vi "CMSClient.vi"() -> ()   [LabVIEW 2013]
uses:
  Controls/CMS Win8 Cluster.ctl
  Controls/CMS Win4 Cluster.ctl
  Controls/DB - Logon Info.ctl
  Controls/DB - Logon Extra Info.ctl
  Controls/Enum - CMS State.ctl
  <vilib>/Utility/miscctls.llb/LVPointTypeDef.ctl
  Controls/CMS Windows Tab.ctl
  Controls/DB - CMS Config WindowView.ctl
  Controls/DB - CMS Execute Active Process.ctl
  Controls/DB - Config WindowView Enum.ctl
  Controls/DB - [Execute].[ActiveProcess] Enum.ctl
  Controls/Global CMS.vi
  <vilib>/Utility/config.llb/Write Key (String).vi
  <vilib>/regexp/Match Regular Expression.xnode
  Controls/Message Code - Enum.ctl
  Controls/Enum - SRTRS State.ctl
  <vilib>/Utility/config.llb/NI_LVConfig.lvlib
panel:
  in  "Tab Footer":enum32{"Page 1"}(tab) caption="Tab Header"
  out "Date Time":string="ver. 13" caption="Plant and Furnace Name"
  in  "Tab Header":enum32{"Page 1"}(tab)
  out "LogoName":picture
  in  "Close":bool
  out "Plant and Furnace Name":string="ver. 13"
  out "ApplicationName":string caption="[LogoName]"
  in  "Tab Body":T1(tab)
  out "Cluster7 WIN8":T2 {"% Hold Complete" scale=0.0..100.0}
  out "Cluster6 WIN8":T2 {"% Hold Complete" scale=0.0..100.0}
  out "Cluster5 WIN8":T2 {"% Hold Complete" scale=0.0..100.0}
  out "Cluster4 WIN8":T2 {"% Hold Complete" scale=0.0..100.0}
  out "Cluster3 WIN8":T2 caption="Cluster3" {"% Hold Complete" scale=0.0..100.0}
  out "Cluster2 WIN8":T2 caption="Cluster2" {"% Hold Complete" scale=0.0..100.0}
  out "Cluster1 WIN8":T2 {"% Hold Complete" scale=0.0..100.0}
  out "Cluster0 WIN8":T2 {"% Hold Complete" scale=0.0..100.0}
  out "Cluster3 WIN4":T3={"Bay"="", "Seq Status"="Waiting to Start", "Record"="", "Hold"="", "% Hold Complete"=0, "Alarm"="", "Temperature"="", "Units"="", "Graph"=[], "Last Updated On"="", "Current Window"=FALSE, "[PlantId.SystemId]"="", "Last Updated (Local)"=""} {"% Hold Complete" scale=0.0..100.0}
  out "Cluster2 WIN4":T3={"Bay"="", "Seq Status"="Waiting to Start", "Record"="", "Hold"="", "% Hold Complete"=0, "Alarm"="", "Temperature"="", "Units"="", "Graph"=[], "Last Updated On"="", "Current Window"=FALSE, "[PlantId.SystemId]"="", "Last Updated (Local)"=""} {"% Hold Complete" scale=0.0..100.0}
  out "Cluster1 WIN4":T3={"Bay"="", "Seq Status"="Waiting to Start", "Record"="", "Hold"="", "% Hold Complete"=0, "Alarm"="", "Temperature"="", "Units"="", "Graph"=[], "Last Updated On"="", "Current Window"=FALSE, "[PlantId.SystemId]"="", "Last Updated (Local)"=""} {"% Hold Complete" scale=0.0..100.0}
  out "Cluster0 WIN4":T3={"Bay"="", "Seq Status"="Waiting to Start", "Record"="", "Hold"="", "% Hold Complete"=0, "Alarm"="", "Temperature"="", "Units"="", "Graph"=[], "Last Updated On"="", "Current Window"=FALSE, "[PlantId.SystemId]"="", "Last Updated (Local)"=""} {"% Hold Complete" scale=0.0..100.0}
  out "Last Updated On":string="2014-10-23 15:23" caption="last updated:"
  out "Key Values":T4={"Recording Duration"=1440.0, "Remaining Hold Time"=1620.0, "Current Temp"=79.84, "Key Values Temperature Units"="°C"} {"Current Temp" format="%#_4f"; "Remaining Hold Time" format="%<%H:%M>t"; "Recording Duration" format="%<%H:%M:%S>t"}
  out "Chart":dynamicdata(graph)
  out "TransactionRunNo (Execute)":string="12" caption="Run No."
  out "cRIO Status":string="DAQ Started. cRIO Simulate Mode." caption="Data Logger"
  out "Transaction No (Execute)":string="110" caption="Transaction No."
  out "% Hold. Time Completed":dbl(slide)=10.0 scale=0.0..100.0
  out "Process Completed":bool
  out "Hold Time Completed":bool
  out "ET3504 Status":string="Program [33]. Segment [Dwell]. Program Status [Running]. ET3500 Simulate Mode." caption="Furnace"
  out "Sequence Status":string="Seq 1/2: +150°C/hr to 80°C & Holding for 00:30 (hh:mm)" caption="Sequence"
  out "Overall Status":bool
  out "WIN1 Bay":string="SRSB-B2"
  in  "MyTab":T5(tab)
  out "Skip Timer Count":i32
  out "WindowView (ORDERed by DB)":string[][](array[string])=[["WIN8", "0", "30", "2", "-1", "0", "4070.SRSB-A1", "4070.SRSB-B2", "4070.SRSB-C3", "4070.SRSB-D4", "4070.SRSB-E5", "4070.SRSB-F6", "4070.SRSB-G7", "4070.SRSB-H8", "", "", "", "", "", "", "", "", "", "", "", ""], ["WIN1", "1", "30", "2", "-1", "0", "4070.SRSB-A1", "4070.SRSB-B2", "4070.SRSB-C3", "4070.SRSB-D4", "4070.SRSB-E5", "", "", "", "", "", "", "", "", "", "", "", "", "", "", ""], ["WIN4", "3", "10", "2", "-1", "0", "4070.SRSB-A1", "4070.SRSB-B2", "", "4070.SRSB-D4", "4070.SRSB-E5", "", "", "", "", "", "", "", "", "", "", "", "", "", "", ""]]
  out "[ToggleWinInterval] Timer":dbl=1.201359748840332 format="%.1g"
  out "[ToggleTabInterval] Timer":dbl=10.53461217880249 format="%.1g"
  out "Current [TabId]":string="WIN8"
  out "[TabId] Index":i32
  out "Time (WIN8 Click)":u32
  out "WIN8 IQ":i32
  out "WIN4 IQ":i32
  out "[ToggleTab] Override":bool=TRUE
  out "[ToggleTab]":bool=TRUE
  out "Page Label when Menu is Clicked":string="WIN8"
  out "New [TabId] Index":i32
  out "Reset [TabId] Index":bool
  out "Stay in [WINDOWxx]":bool
  out "[WINDOWxx] Stay":string="4070.SRSB-A1"
  out "[WINDOWxx]":string="4070.SRSB-C3"
  out "Empty [WINDOWxx]":string[](array[string])
  out "Skip WIN Timer":bool=TRUE
  out "Skip TAB Timer":bool=TRUE
  out "Current WindowView":string[](array[string])
  out "# of requested Windowxx":i32
  out "Property Node":errorcluster
  out "Load History":errorcluster
  out "Cluster0 WIN1":T2={"Bay"="", "Seq Status"="Waiting to Start", "Record"="", "Hold"="", "% Hold Complete"=0, "Alarm"="", "Temperature"="", "Units"="", "Graph"=[], "Last Updated On"="", "Current Window"=FALSE, "[PlantId.SystemId]"="", "Last Updated (Local)"=""} {"% Hold Complete" scale=0.0..100.0}
  out "SubPanel Error":errorcluster
  out "Logon OK":bool
  in  "[TabUserAccess]":bool[](array[boolean])=[FALSE, FALSE, FALSE, FALSE, FALSE, FALSE, FALSE, FALSE, FALSE, FALSE, FALSE, FALSE, FALSE, FALSE, FALSE, FALSE, FALSE, FALSE, FALSE, FALSE]
  in  "Logon Extra":T6
  in  "Logon":T7
  out "Current VI's path":path=path "C:/Users/CK/workspace/LabVIEW/Stress Relief Temperature Recording/VIs/CMSClient.vi"
  out "Front Panel Window:State":T8(ring)=enum."Closed"
  out "Execution:State":T9(ring)=enum."Idle"
  out "Admin User UI":refnum<vi>
  out "Logon UI":refnum<vi>
  out "Config UI":refnum<vi>
  in  "Application":string="CMS"
  out "ini File":errorcluster
  out "LogonName Error":errorcluster
  out "[ToggleTabInterval]":dbl=10.0 format="%#_13g"
  out "Min [ToggleWinInterval]":i32=2
  out "Station":string="C001"
  out "Plant":string="4070"
  out "[ToggleWinInterval]":dbl=2.0 format="%#_13g"
  out "Min [ToggleTabInterval]":i32=10
  out "LabVIEW Directory Path":path=path "C:/Program Files (x86)/National Instruments/LabVIEW 2013"
  out "Application:Name":string="LabVIEW.exe"
  out "[TimeZone] (Plant)":string="+8"
  out "[CmsServerTz] (CMS)":string="+7"
  out "TimeZone Diff (NA)":i32=-1
  out "Time Offset":dbl=-0.44188642501831055
  out "Plant and Furnace Name (B4 Logon)":string="ver. 13" caption="Plant and Furnace Name"
  out "DisplayDurationInMin":i32=60
  out "Error Out":errorcluster
  out "Show Debug TAB":bool=TRUE caption="Show Debug Tab"
  out "Lite Version":bool
  out "Quit Flag":bool=TRUE
  out "Close Flag":bool=TRUE
  out "WIN8 Array":refnum<vi>[](array[refnum])
  out "WIN4 Array":refnum<vi>[](array[refnum])
  in  "PlantId.SystemId - Last Updated (Local)":string[][](array[string])
  out "MHandler":errorcluster
  out "DB":errorcluster
  in  "DB - Logon":bool=TRUE
  out "File Version":string="ver. 13.0f1"
  in  "Debug Close":bool caption="Close"
  # "Process Status"
  # "System Status"
  # "(hh:mm:ss)"
  # "(hh:mm)"
  # "User Details"
  # "System Status"
  # "Logon"
  # "2014-10-21 15:01\n[TabId],                         w.[IsDefault],        v.[ToggleTabInterval],w.[ToggleWinInterval], v.[ToggleTab],        v.[DisplayPlant],       w.[Window01],            w.[Window02]"
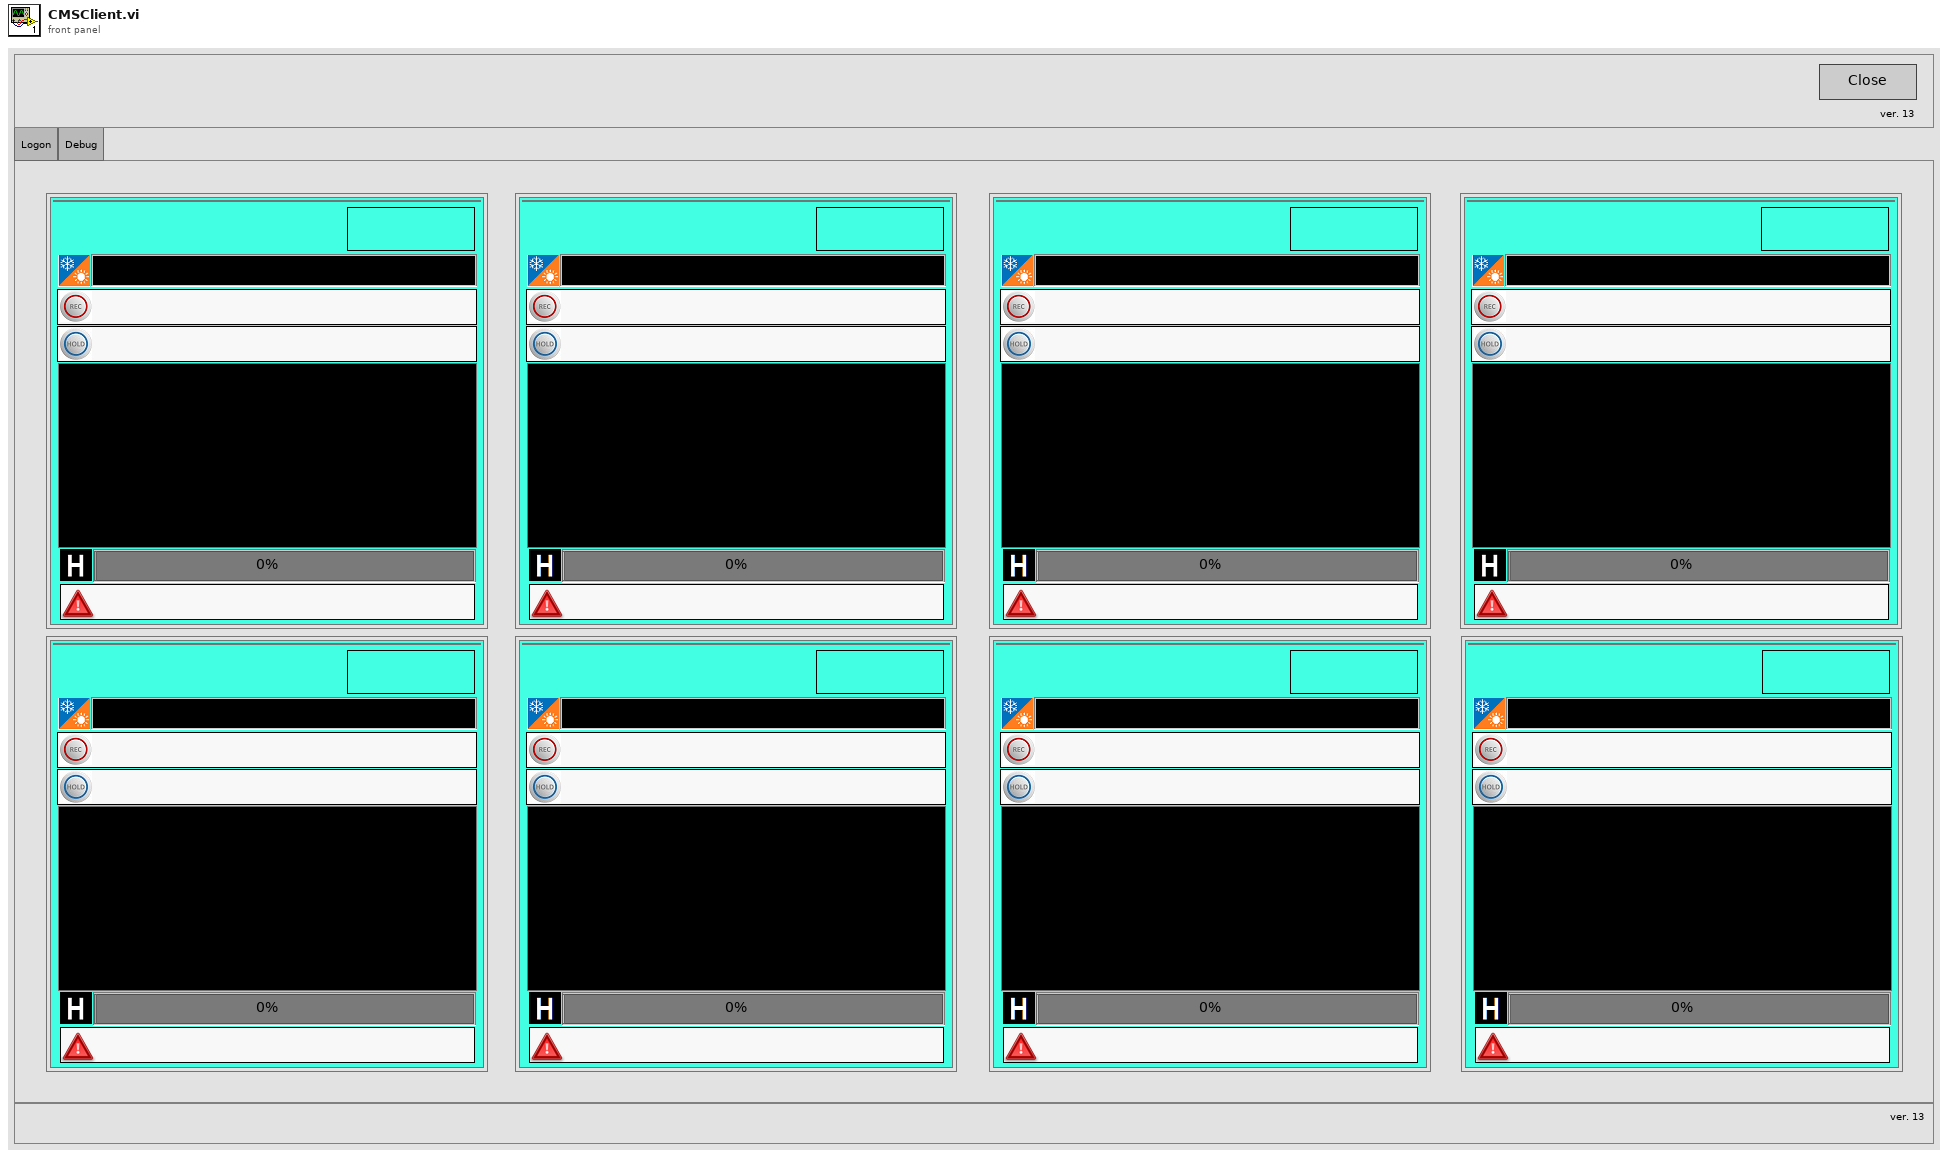
[diagram p1: front panel]
types:
  T1 = enum32{"WIN8", "WIN4", "WIN1", "Admin", "Config", "Logon", "Debug"}
  T2 = typedef "CMS Win8 Cluster.ctl" = cluster{"Bay":string, "Seq Status":string, "Record":string, "Hold":string, "% Hold Complete":u8, "Alarm":string, "Temperature":string, "Units":string, "Graph":dbl[][], "Last Updated On":string, "Current Window":bool, "[PlantId.SystemId]":string, "Last Updated (Local)":string}
  T3 = typedef "CMS Win4 Cluster.ctl" = cluster{"Bay":string, "Seq Status":string, "Record":string, "Hold":string, "% Hold Complete":u8, "Alarm":string, "Temperature":string, "Units":string, "Graph":dbl[][], "Last Updated On":string, "Current Window":bool, "[PlantId.SystemId]":string, "Last Updated (Local)":string}
  T4 = cluster{"Recording Duration":dbl, "Remaining Hold Time":dbl, "Current Temp":dbl, "Key Values Temperature Units":string}
  T5 = enum32{"WindowView", "Single Window", "SubPanel", "Settings", "Others", "DB"}
  T6 = typedef "DB - Logon Extra Info.ctl" = cluster{"Plant Name":string, "UserName":string, "Hostname [ClientName]":string, "IsUnicode":bool}
  T7 = typedef "DB - Logon Info.ctl" = cluster{"PlantID":string, "SystemID":string, "UserID":string, "DomainID":string, "LanguageID":string, "StationID":string}
  T8 = enum32{"Invalid", "Standard", "Closed", "Hidden", "Minimized", "Maximized"}
  T9 = enum32{"Bad", "Idle", "Run top level", "Running"}
  T10 = typedef "Enum - CMS State.ctl" = enum16{"READY TO START", "RUNNING Process", "QUIT"}
  T11 = enum16{"Always On", "Always Off", "Off While Running"}
  T12 = typedef "CMS Windows Tab.ctl" = enum32{"WIN8", "WIN4", "WIN1", "Admin", "Config", "Logon", "Debug"}
  T13 = typedef "LVPointTypeDef.ctl" = cluster{"Horizontal":i16, "Vertical":i16}
  T14 = enum8{"Enabled", "Disabled", "Disabled and Grayed Out"}
  T15 = cluster{"LogoFile":string, "Software Solution Name":string}
  T16 = typedef "Connection Information Cluster.ctl" = cluster{"Connection ":string, "Username":string, "Password":string}
  T17 = cluster{"Show LabVIEW Error":bool, "Show Debug Tab":bool, "Show Scrollbars":bool, "ToggleTab":bool}
  T18 = typedef "imagedata.ctl" = cluster{"image type":i32, "image depth":i32, "image":u8[], "mask":u8[], "colors":u32[], "Rectangle":cluster{"left":i16, "top":i16, "right":i16, "bottom":i16}}
  T19 = typedef "Enum - SRTRS State.ctl" = enum16{"READY TO START", "START Recipe", "START Recovery", "BEGIN Process", "RUNNING Process", "END Process", "Spare Enum", "END Recipe", "ERROR Handling", "QUIT"}
  T20 = typedef "DB - CMS Config WindowView.ctl" = enum16{"SELECT [Config].[View]"}
  T21 = typedef "DB - Config WindowView Enum.ctl" = enum16{"w.[TabId]", "w.[Number]", "w.[ToggleTabInterval]", "w.[ToggleWinInterval]", "v.[ToggleTab]", "v.[DisplayPlant]", "w.[Window01]", "w.[Windowxx]"}
  T22 = typedef "DB - CMS Execute Active Process.ctl" = enum16{"INSERT INTO [Execute].[ActiveProcess]", "UPDATE [Execute].[ActiveProcess]", "SELECT [Execute].[ActiveProcess]", "UPDATE FILESTREAM", "SELECT FILESTREAM", "Check [IsActive]"}
  T23 = typedef "DB - [Execute].[ActiveProcess] Enum.ctl" = enum16{"[IsActive]", "[TransactionNo]", "[TransactionRunNo]", "[SequenceStatus]", "[StartRecordTime]", "[EndRecordTime]", "[StartHoldTime]", "[EndHoldTime]", "[Message1]", "[Message2]", "[HoldTimeRemaining]", "[HoldTimePercentage]", "[HoldProgressColor]", "[OrderNumbers]", "[CurrentTemp]", "[UnitOfTemperature]", "[IsAppClientLive]", "[RawDataFile]", "[RecordedMinutes]", "[FurnaceControlStatus]", "[FurnaceControlColor]", "[ControllerStatus]", "[ControllerColor]", "[IsControllerOnline]", "[ProcessColor]", "[OverallColor]", "[LastUpdatedOn]", "[LastUpdatedCmsTime]", "[Inactive]"}
  T24 = enum16{"INSERT INTO [Execute].[ActiveProcess]", "UPDATE [Execute].[ActiveProcess]", "SELECT [Execute].[ActiveProcess]", "UPDATE FILESTREAM", "SELECT FILESTREAM"}
  T25 = typedef "NI_LVConfig.lvlib/Config Data RefNum.ctl" = refnum<k1>
  T26 = typedef "Message Code - Enum.ctl" = enum16{"<APP><I 100>", "<APP><E 101>", "<APP><I 110>", "<APP><W 111>", "<APP><I 112>", "<APP><W 113>", "<APP><I 114>", "<APP><I 115>", "<APP><I 116>", "<APP><W 117>", "<APP><I 120>", "<APP><W 121>", "<APP><E 122>", "<APP><W 130>", "<APP><W 131>", "<APP><W 132>", "<APP><W 133>", "<APP><W 134>", "<DB><I 150>", "<DB><I 151>", "<DB><W 152>", "<APP><I 200>", "<APP><I 201>", "<APP><W 202>", "<APP><E 203>", "<DB><I 300>", "<DB><I 301>", "<DB><W 302>", "<DB><I 305>", "<DB><I 306>", "<DB><W 307>", "<DB><W 310>", "<cRIO><I 400>", "<cRIO><W 401>", "<cRIO><I 402>", "<cRIO><W 403>", "<ET><I 500>", "<ET><W 501>", "<ET><I 600>", "<ET><W 601>", "<ET><E 602>", "<ET><I 610>", "<ET><W 611>", "<ET><E 612>"}
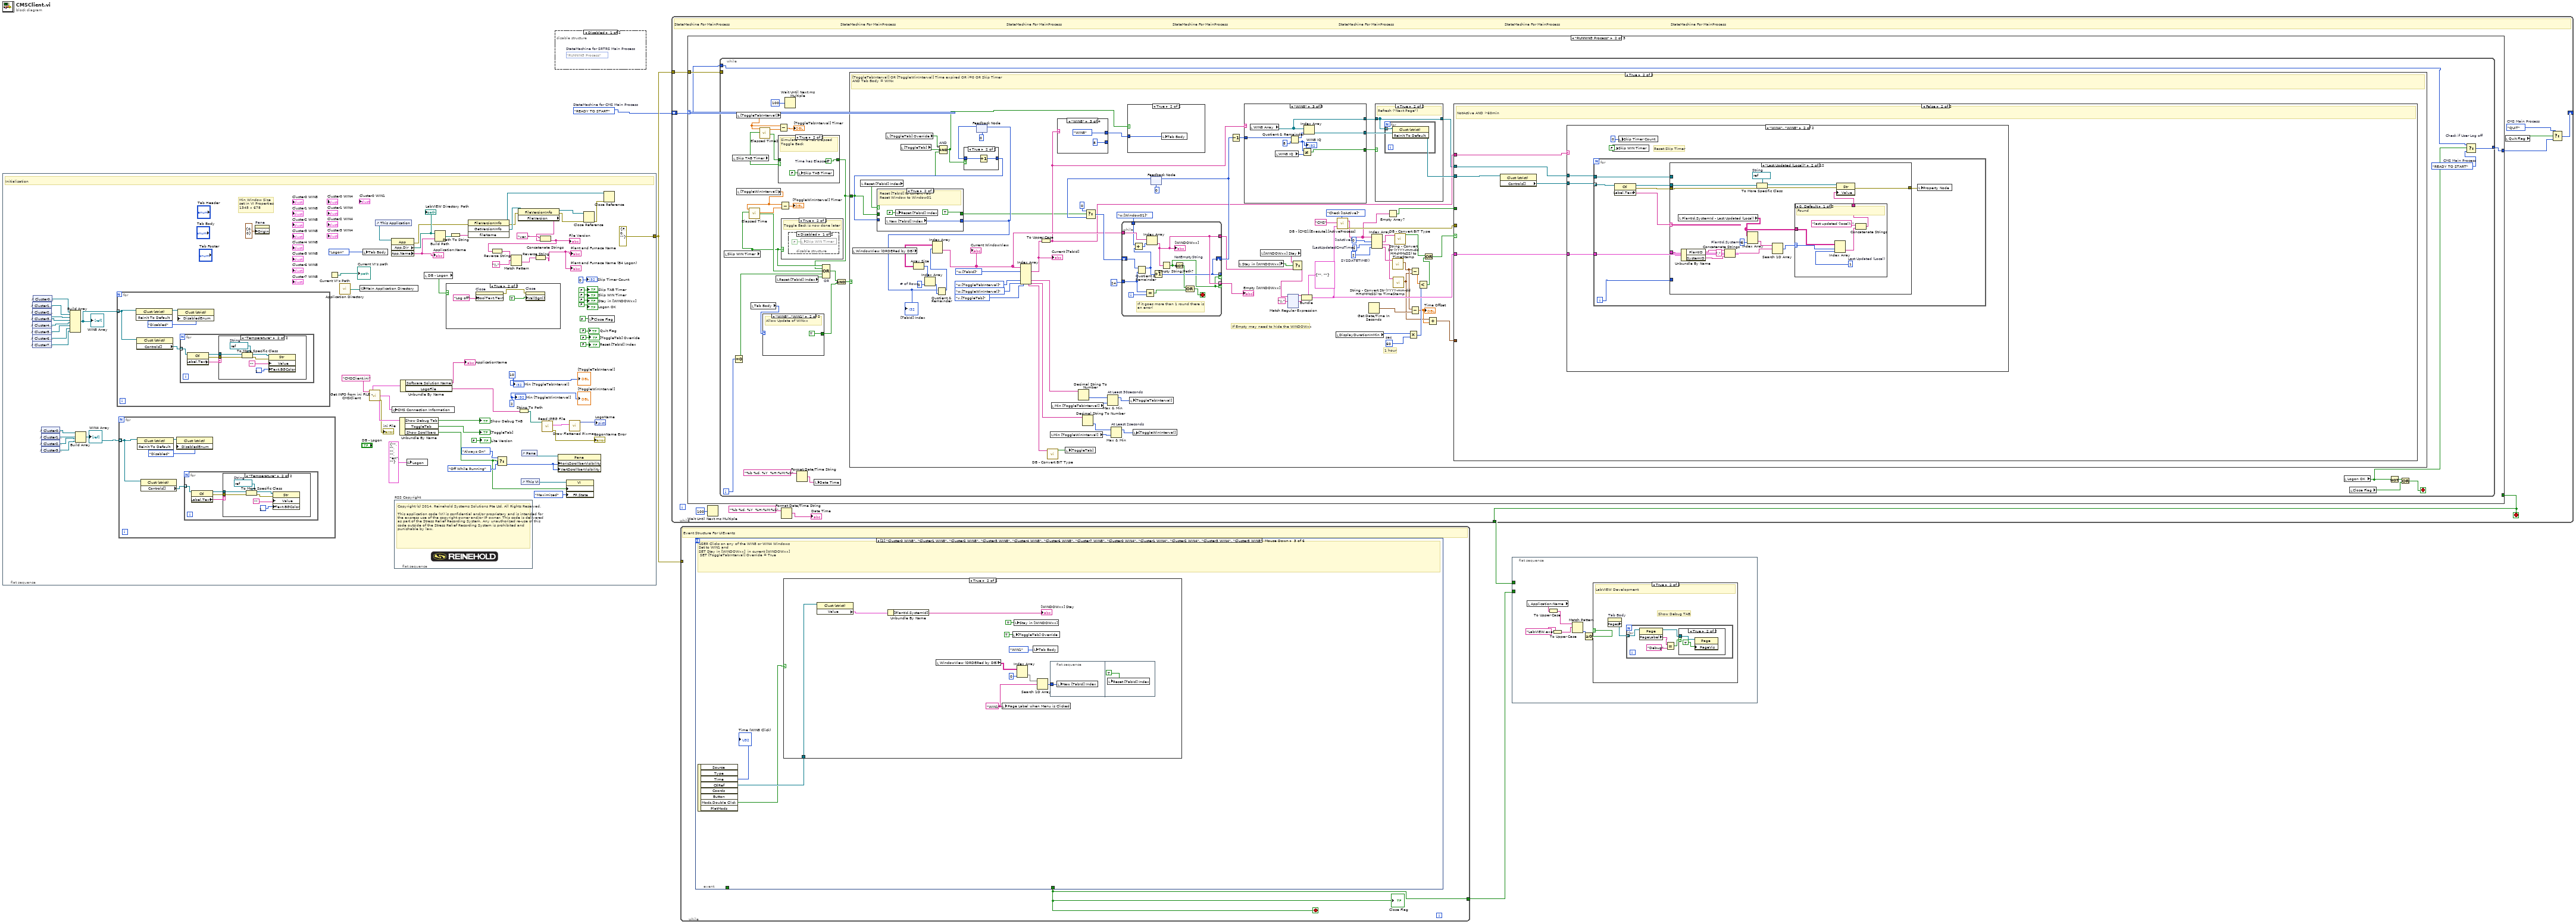
[diagram p0: block diagram]
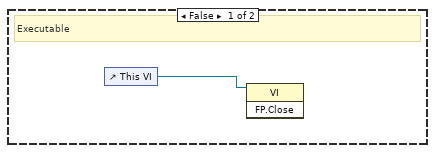
[diagram p2: hidden frame]
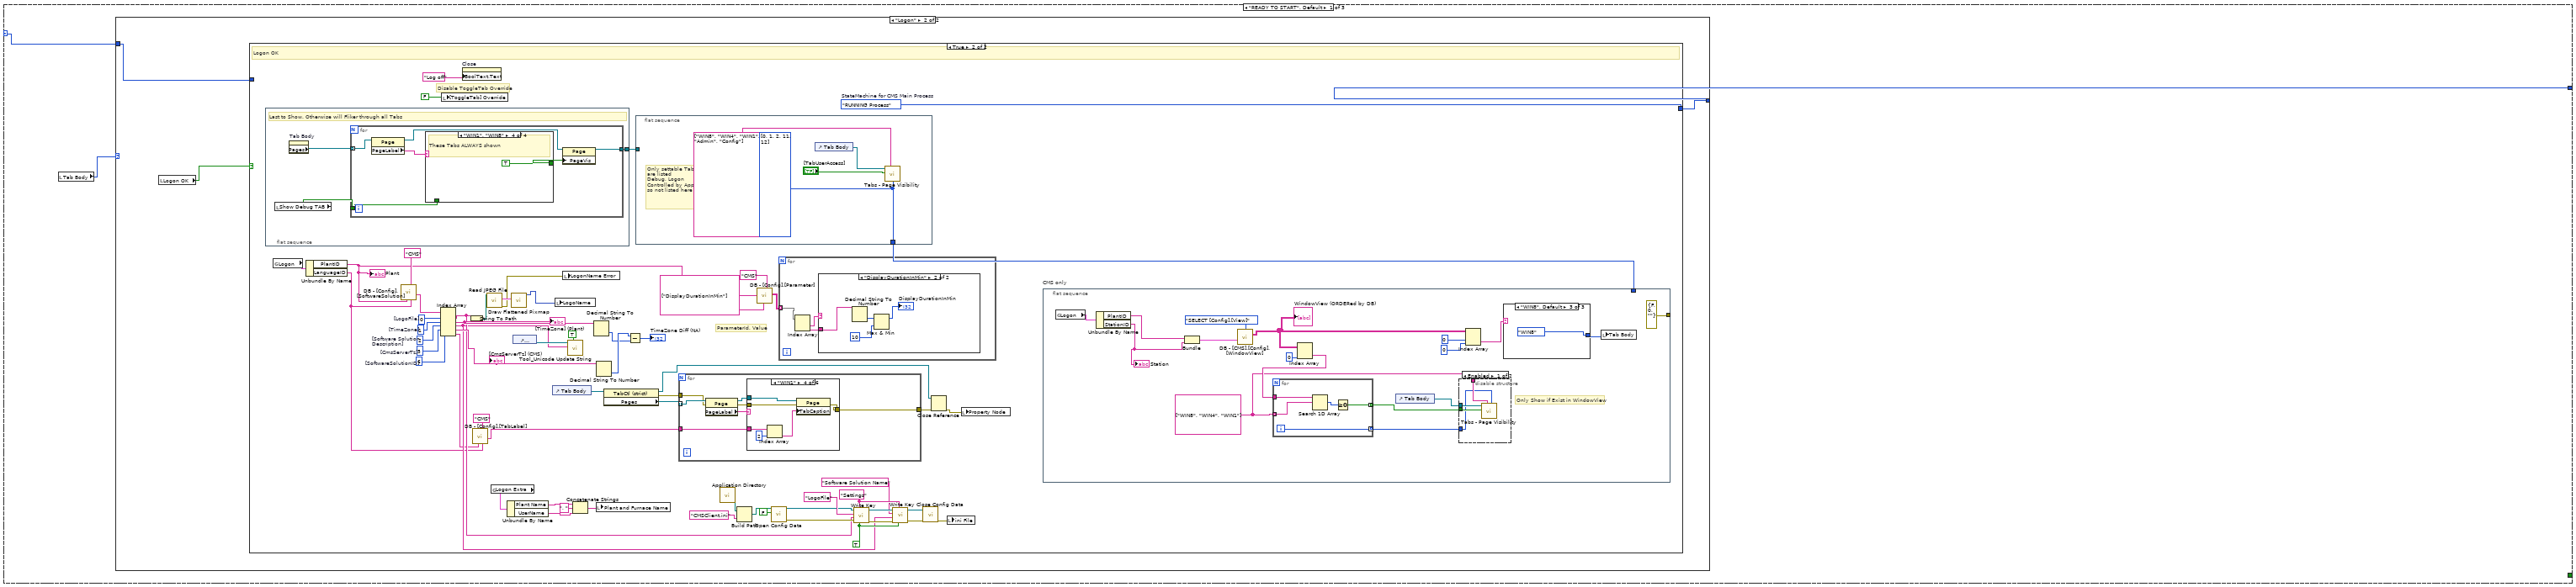
[diagram p5: hidden frame]
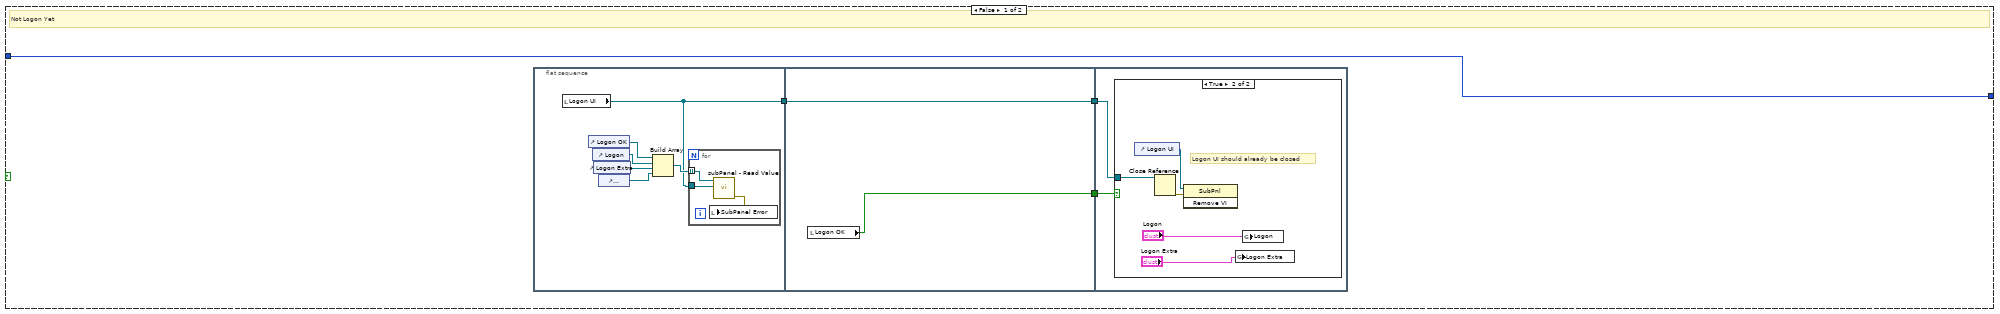
[diagram p7: hidden frame]
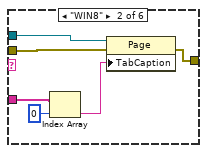
[diagram p11: hidden frame]
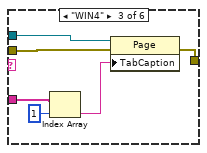
[diagram p12: hidden frame]
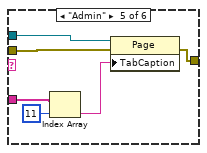
[diagram p13: hidden frame]
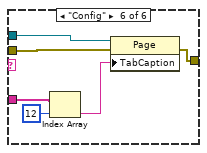
[diagram p14: hidden frame]
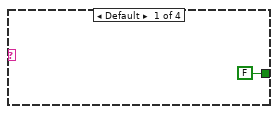
[diagram p15: hidden frame]
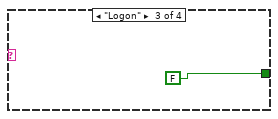
[diagram p17: hidden frame]
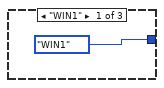
[diagram p19: hidden frame]
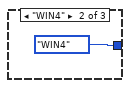
[diagram p20: hidden frame]
diagram:
  w3 = Enum_-_CMS_State."READY TO START"  # StateMachine for CMS Main Process
  n1 = flat-sequence {
    tunnel: [errorcluster {"status"=FALSE, "code"=0, "source"=""} ("error constant")] -> w4
    frame #0 {
      w8 = 2
      w9 = 10
      # "Min Window Size\nset in VI Properties\n1345 x 678"
      # "Initialisation"
      n2 = control-ref of="Cluster1 WIN8"() -> (w67:refnum<vi>)
      n3 = control-ref of="Cluster2 WIN8"() -> (w68:refnum<vi>)
      n4 = control-ref of="Cluster3 WIN8"() -> (w69:refnum<vi>)
      n5 = control-ref of="Cluster4 WIN8"() -> (w70:refnum<vi>)
      n6 = control-ref of="Cluster5 WIN8"() -> (w71:refnum<vi>)
      n7 = control-ref of="Cluster6 WIN8"() -> (w72:refnum<vi>)
      n8 = control-ref of="Cluster7 WIN8"() -> (w73:refnum<vi>)
      n9 = control-ref of="Cluster0 WIN8"() -> (w61:refnum<vi>)
      n10 = control-ref of="Cluster0 WIN4"() -> (w65:refnum<vi>)
      n11 = control-ref of="Cluster1 WIN4"() -> (w64:refnum<vi>)
      n12 = control-ref of="Cluster2 WIN4"() -> (w63:refnum<vi>)
      n13 = control-ref of="Cluster3 WIN4"() -> (w62:refnum<vi>)
      n14 = Build Array(w61, w67, w68, w69, w70, w71, w72, w73) -> (w66:refnum<vi>[])
      "WIN8 Array" <- w66
      n15 = Build Array(w65, w64, w63, w62) -> (w32:refnum<vi>[])
      "WIN4 Array" <- w32
      n16 = for {
        tunnel: w66 -> [w96] mode=indexing
        n17 = invoke class="Clust (strict)" method="Reinit To Default"(reference=w96) -> (reference out=w98:refnum<vi>)  [unwired: 2 in, 2 out]
        n18 = property class="Clust (strict)"(reference=w96) -> ("Controls[]"=w95:refnum<vi>[])  [unwired: 1 in, 2 out]
        n19 = property class="Clust (strict)"(reference=w98, "DisabledEnum"=T14."Disabled" ("Disabled")) -> ()  [unwired: 1 in, 2 out]
        n20 = for {
          tunnel: w95 -> [w100] mode=indexing
          n21 = property class="Ctl"(reference=w100) -> (reference out=w102:refnum<vi>, error out=w101:errorcluster, "Label.Text"=w99:string)  [unwired: 1 in]
          n22 = case shown="\"Temperature\"" w99 {
            tunnel: w102 -> [_ w108]
            tunnel: w101 -> [_ w107]
            frame "False", Default {
            }
            frame "Temperature" {
              w109 = refnum<vi> refnum  # String
              n23 = To More Specific Class(target class=w109, reference=w108, error in=w107) -> (specific class reference=w105:refnum<vi>, error out=w106:errorcluster)
              n24 = property class="Str"(reference=w105, error in=w106, "Value"="", "Text.BGColor"=u32 16777216) -> ()  [unwired: 2 out]
            }
          }
        }
      }
      n25 = for {
        tunnel: w32 -> [w78] mode=indexing
        n26 = invoke class="Clust (strict)" method="Reinit To Default"(reference=w78) -> (reference out=w80:refnum<vi>)  [unwired: 2 in, 2 out]
        n27 = property class="Clust (strict)"(reference=w78) -> ("Controls[]"=w77:refnum<vi>[])  [unwired: 1 in, 2 out]
        n28 = property class="Clust (strict)"(reference=w80, "DisabledEnum"=T14."Disabled" ("Disabled")) -> ()  [unwired: 1 in, 2 out]
        n29 = for {
          tunnel: w77 -> [w82] mode=indexing
          n30 = property class="Ctl"(reference=w82) -> (reference out=w84:refnum<vi>, error out=w83:errorcluster, "Label.Text"=w81:string)  [unwired: 1 in]
          n31 = case shown="\"Temperature\"" w81 {
            tunnel: w84 -> [_ w90]
            tunnel: w83 -> [_ w89]
            frame "False", Default {
            }
            frame "Temperature" {
              w91 = refnum<vi> refnum  # String
              n32 = To More Specific Class(target class=w91, reference=w90, error in=w89) -> (specific class reference=w87:refnum<vi>, error out=w88:errorcluster)
              n33 = property class="Str"(reference=w87, error in=w88, "Value"="", "Text.BGColor"=u32 16777216) -> ()  [unwired: 2 out]
            }
          }
        }
      }
      n34 = property on="Pane" class="Pane"("Origin"=T13 {"Horizontal"=0, "Vertical"=0}) -> ()  [unwired: 2 in, 2 out]
      n35 = Current VI's Path() -> (path=→"Current VI's path":path)
      n36 = call <vilib>:"Application Directory.vi"() -> ("Application Directory"=w24:path)
      n37 = global write "Global CMS.vi" "Main Application Directory"(w24) -> ()
      n38 = local write "Tab Body"(CMS_Windows_Tab."Logon" ("Tab Body")) -> ()
      n39 = call "Get INFO from ini FILE - CMSClient.vi"("ini Name"="CMSClient.ini") -> ("Settings"=w54:T15, "CMS Connection Information"=w55:T16, "Settings Boolean"=w56:T17, "Error Out"=→"ini File":errorcluster)  [unwired: 8 in, 3 out]
      n40 = control-ref of="This Application"() -> (w46:refnum<vi>)
      n41 = property class="App"(reference=w46) -> (error out=w39:errorcluster, "App.Dir"=w45:path, "App.Name"=w33:string)  [unwired: 1 in, 1 out]
      "LabVIEW Directory Path" <- w45
      "Application:Name" <- w33
      n42 = global write "Global CMS.vi" "CMS Connection Information"(w55) -> ()
      n43 = flat-sequence "RSS Copyright" {
        frame #0 {
          # "Copyright (c) 2014, Reinehold Systems Solutions Pte Ltd. All Rights Reserved.\n\nThis application code (VI) is confidential and/or proprietary and is intended for the express use of the copyright owner and/or IP owner. This code is delivered as part of the Stress Relief Recording System. Any unauthorized re-use of this code outside of the Stress Relief Recording System is prohibited and punishable by law."
        }
      }
      n44 = Unbundle By Name(w56) -> ("Show Debug Tab"=→"Show Debug TAB":bool, "ToggleTab"=→"[ToggleTab]":bool, "Show Scrollbars"=w17:bool)
      n45 = Unbundle By Name(w54) -> ("Software Solution Name"=→"ApplicationName":string, "LogoFile"=w14:string)
      n46 = global write "Global CMS.vi" "Logon"(T7 {"PlantID"="", "SystemID"="", "UserID"="", "DomainID"="", "LanguageID"="en", "StationID"=""} ("Logon")) -> ()
      n47 = local read "DB - Logon"() -> (w59:bool)
      n48 = Build Path(base path=w45, name or relative path=w33) -> (appended path=w44:path)
      n49 = case shown="True" w59 {
        frame False {
        }
        frame True {
          n50 = property on="Close" class="Bool (strict)"("BoolText.Text"="Log off" ("Label.Text")) -> (error out=w92:errorcluster)  [unwired: 2 in, 1 out]
          n51 = property on="Close" class="Bool (strict)"(error in=w92, "Val(Sgnl)"=TRUE ("Value (Signaling)")) -> ()  [unwired: 1 in, 2 out]
        }
      }
      n52 = Path To String(path=w44) -> (string=w43:string)
      n53 = invoke class="FileVersionInfo" method="GetVersionInfo"(error in=w39, "fileName"=w43) -> (reference out=w40:refnum<k24>, error out=w38:errorcluster, "GetVersionInfo"=w42:refnum<k24>)  [unwired: 2 in, 1 out]
      n54 = Select(t=T11."Always On" ("Horizontal Scrollbar Visibility"), s=w17, f=T11."Off While Running" ("Horizontal Scrollbar Visibility")) -> (s? t:f=w20:T11)
      n55 = property class="FileVersionInfo"(reference=w42, error in=w38) -> (reference out=w41:refnum<k24>, error out=w37:errorcluster, "FileVersion"=w34:string)
      n56 = String To Path(string=w14) -> (path=w13:path)
      n57 = control-ref of="This VI"() -> (w18:refnum<vi>)
      n58 = control-ref of="Pane"() -> (w19:refnum<vi>)
      n59 = Concatenate Strings("ver. ", w34) -> (w28:string)
      "File Version" <- w28
      n60 = Reverse String(1:w28) -> (0:w29:string)
      n61 = Match Pattern(string=w29, regular expression="\\." ("search string")) -> (after substring=w31:string)  [unwired: 1 in, 3 out]
      n62 = Reverse String(1:w31) -> (0:→"Plant and Furnace Name" →"Plant and Furnace Name (B4 Logon)":string)
      n63 = call <vilib>:"Read JPEG File.vi"("path to JPEG file"=w13) -> ("error out"=→"LogonName Error":errorcluster, "image data"=w15:T18)  [unwired: 8 in, 1 out]
      n64 = property class="Pane"(reference=w19, "HorizScrollbarVisibility"=w20, "VertScrollbarVisibility"=w20) -> ()  [unwired: 1 in, 2 out]
      n65 = property class="VI"(reference=w18, "Front Panel.TitleBarVis"=w17, "FP.State"=T8."Maximized" ("Front Panel Window:State")) -> ()  [unwired: 1 in, 2 out]
      n66 = call <vilib>:"Draw Flattened Pixmap.vi"("image data"=w15) -> ("new picture"=→"LogoName":picture)  [unwired: 8 in]
      n67 = Close Reference(reference=w41, error in (no error)=w37) -> (error out=w36:errorcluster)
      n68 = local write "Close Flag"(FALSE ("Close Flag")) -> ()
      n69 = Close Reference(reference=w40, error in (no error)=w36) -> ()  [unwired: 1 out]
      "Logon OK" <- FALSE ("Logon OK")
      "Quit Flag" <- FALSE ("Quit Flag")
      "Lite Version" <- FALSE ("Lite Version")
      "Min [ToggleWinInterval]" <- w8
      "[ToggleTabInterval]" <- w9
      "Min [ToggleTabInterval]" <- w9
      "[ToggleWinInterval]" <- w8
      "[ToggleTab] Override" <- FALSE ("[ToggleTab] Previous State")
      "Reset [TabId] Index" <- FALSE ("Reset [TabId] Index")
      "Stay in [WINDOWxx]" <- FALSE ("Stay in [WINDOWxx]")
      "Skip WIN Timer" <- FALSE ("Skip Timer")
      "Skip TAB Timer" <- FALSE ("Skip Timer 2")
      "Skip Timer Count" <- 0 ("Skip Timer Count")
    }
  }
  n70 = disable-structure shown="Disabled" {
    frame Disabled {
      (unwired) Enum_-_SRTRS_State."RUNNING Process"  # StateMachine for SRTRS Main Process
    }
    frame Enabled {
    }
  }
  n71 = while {
    tunnel: w4 -> [w119]
    shift-right: [w115] -> _
    shift-left: w3 -> [w118]
    tunnel: [w112] -> w2
    stop <- w112 stop-if-true
    w116 = Enum_-_CMS_State."QUIT"  # CMS Main Process
    # "StateMachine For MainProcess                                                                                             StateMachine For MainProcess                                                                                             StateMachine For MainProcess                                                                                             StateMachine For MainProcess                                                                                             StateMachine For MainProcess                                                                                             StateMachine For MainProcess                                                                                             StateMachine For MainProcess"
    n72 = case shown="\"RUNNING Process\"" w118 {
      selector: w118 -> [w120 w301 w1178]
      tunnel: w119 -> [_ w302 _]
      tunnel: [_ _ TRUE] -> w112
      tunnel: [w121 w300 w1178] -> w114
      frame "READY TO START", Default {
        n73 = local read "Tab Body"() -> (w122:T1)
        n74 = case shown="\"Logon\"" w122 {
          tunnel: [w123 w125] -> w121
          tunnel: w120 -> [w123 w124]
          frame "WIN8", Default {
          }
          frame "Logon" {
            n75 = local read "Logon OK"() -> (w126:bool)
            n76 = case shown="True" w126 {
              tunnel: [w127 w208] -> w125
              tunnel: w124 -> [w127 _]
              frame False {
                # "Not Logon Yet"
                n77 = flat-sequence {
                  tunnel: [w132] -> w128
                  tunnel: [w141] -> w130
                  tunnel: [w140] -> w129
                  tunnel: w128 -> [w140]
                  tunnel: w130 -> [w143]
                  tunnel: w129 -> [w142]
                  frame #0 {
                    n78 = local read "Logon UI"() -> (w132:refnum<vi>)
                    n79 = control-ref of="Logon OK"() -> (w131:refnum<vi>)
                    n80 = control-ref of="Logon"() -> (w135:refnum<vi>)
                    n81 = control-ref of="Logon Extra"() -> (w134:refnum<vi>)
                    n82 = control-ref of="[TabUserAccess]"() -> (w133:refnum<vi>)
                    n83 = Build Array(w131, w135, w134, w133) -> (w136:refnum<vi>[])
                    n84 = for {
                      tunnel: w132 -> [w139]
                      tunnel: w136 -> [w138] mode=indexing
                      n85 = call "subPanel - Read Value.vi"("subPanel Ref"=w139, "CtlRef"=w138) -> ("Error Out"=w137:errorcluster)  [unwired: 6 in, 3 out]
                      n86 = local write "SubPanel Error"(w137) -> ()
                    }
                  }
                  frame #1 {
                    n87 = local read "Logon OK"() -> (w141:bool)
                  }
                  frame #2 {
                    n88 = case shown="True" w143 {
                      tunnel: w142 -> [_ w147]
                      frame False {
                      }
                      frame True {
                        # "Logon UI should already be closed"
                        n89 = control-ref of="Logon UI"() -> (w146:refnum<vi>)
                        n90 = Close Reference(reference=w147) -> (error out=w148:errorcluster)  [unwired: 1 in]
                        n91 = invoke on="Invoke Node" class="SubPnl" method="Remove VI"(reference=w146, error in=w148) -> ()  [unwired: 1 in, 3 out]
                        n92 = global write "Global CMS.vi" "Logon Extra"("Logon Extra") -> ()
                        n93 = global write "Global CMS.vi" "Logon"("Logon") -> ()
                      }
                    }
                  }
                }
              }
              frame True {
                w160 = 6  # [SoftwareSolutionID]
                w170 = TRUE ("write raw string? (F)")
                w169 = "Settings" ("section")
                w198 = 5  # [CmsServerTz]
                w205 = 1  # [TimeZone]
                w204 = 2  # [Software Solution Description]
                w203 = 0  # [LogoFile]
                w208 = Enum_-_CMS_State."RUNNING Process"  # StateMachine for CMS Main Process
                # "ParameterId, Value"
                # "Disable ToggleTab Override"
                # "Logon OK"
                n94 = flat-sequence {
                  tunnel: [w254] -> w186
                  frame #0 {
                    # "Last to Show. Otherwise will Fliker through all Tabs"
                    n95 = local read "Show Debug TAB"() -> (w255:bool)
                    n96 = property on="Tab Body" class="TabCtl (strict)"() -> ("Pages"=w256:refnum<vi>[])  [unwired: 2 in, 2 out]
                    n97 = for {
                      tunnel: w256 -> [w262] mode=indexing
                      tunnel: w255 -> [w261]
                      tunnel: [w257] -> w254
                      n98 = property class="Page"(reference=w262) -> (reference out=w258:refnum<vi>, "PageLabel"=w260:string)  [unwired: 1 in, 1 out]
                      n99 = case shown="\"WIN1\", \"WIN8\"" w260 {
                        tunnel: w261 -> [_ w264 _ _]
                        tunnel: [FALSE ("Show Debug TAB") w264 FALSE TRUE] -> w259
                        frame Default {
                        }
                        frame "Debug" {
                          # "Debug dependent of \n\"Show Report Tab ONLY\""
                        }
                        frame "Logon" {
                        }
                        frame "WIN1", "WIN8" {
                          # "These Tabs ALWAYS shown"
                        }
                      }
                      n100 = property class="Page"(reference=w258, "PageVis"=w259) -> (reference out=w257:refnum<vi>)  [unwired: 1 in, 1 out]
                    }
                  }
                }
                n101 = global read "Global CMS.vi" "Logon"() -> (w185:T7)
                n102 = Unbundle By Name(w185) -> ("PlantID"=w162:string, "LanguageID"=w158:string)
                "Plant" <- w162
                n103 = call "DB - [Config].[SoftwareSolution].vi"("[LanguageId]"=w158, "Application"="CMS", "[PlantId]"=w162) -> ("1D data"=w202:string[])  [unwired: 6 in, 2 out]
                n104 = Index Array(array=w202, index #1=w203, index #2=w205, index #3=w204, index #4=w198, index #5=w160) -> (element #1=w171:string, element #2=w197:string, element #3=w167:string, element #4=w196:string, element #5=w159:string)
                "[TimeZone] (Plant)" <- w197
                "[CmsServerTz] (CMS)" <- w196
                n105 = local write "[ToggleTab] Override"(FALSE ("[ToggleTab] Override")) -> ()
                n106 = property on="Close" class="Bool (strict)"("BoolText.Text"="Log off") -> ()  [unwired: 2 in, 2 out]
                n107 = String To Path(string=w171) -> (path=w201:path)
                n108 = call "DB - [Config].[TabLabel].vi"("[LanguageId]"=w158, "Application"="CMS", "[SolutionId]"=w159) -> ("1D data"=w153:string[])  [unwired: 6 in, 2 out]
                n109 = call <vilib>:"Read JPEG File.vi"("path to JPEG file"=w201) -> ("error out"=w181:errorcluster, "image data"=w200:T18)  [unwired: 8 in, 1 out]
                n110 = global read "Global CMS.vi" "Logon Extra"() -> (w191:T6)
                n111 = Unbundle By Name(w191) -> ("Plant Name"=w190:string, "UserName"=w188:string)
                n112 = call <vilib>:"Draw Flattened Pixmap.vi"("image data"=w200) -> ("new picture"=w182:picture)  [unwired: 8 in]
                n113 = control-ref of="ApplicationName"() -> (w184:refnum<vi>)
                n114 = control-ref of="Tab Body"() -> (w156:refnum<vi>)
                n115 = local write "LogoName"(w182) -> ()
                n116 = local write "LogonName Error"(w181) -> ()
                n117 = call "Tool_Unicode Update String.vi"("Interpret as Unicode (T)"=TRUE, "String Value"=w167, "String Control Reference"=w184) -> ()  [unwired: 5 in, 2 out]
                n118 = Concatenate Strings(w190, ", " ("string"), w188) -> (w187:string)
                n119 = Decimal String To Number(string=w197) -> (number=w194:i32)  [unwired: 2 in, 1 out]
                n120 = local write "Plant and Furnace Name"(w187) -> ()
                n121 = Decimal String To Number(string=w196) -> (number=w195:i32)  [unwired: 2 in, 1 out]
                n122 = property class="TabCtl (strict)"(reference=w156) -> (reference out=w152:refnum<vi>, error out=w154:errorcluster, "Pages"=w155:refnum<vi>[])  [unwired: 1 in]
                n123 = Subtract(x=w195, y=w194) -> (x-y=→"TimeZone Diff (NA)":i32)
                n124 = flat-sequence {
                  tunnel: [w296] -> w206
                  tunnel: w186 -> [_]
                  frame #0 {
                    w296 = i32[] [0, 1, 2, 11, 12] ("Matching Tab#")
                    # "Only settable Tabs\nare listed\nDebug, Logon\nControlled by App\nso not listed here"
                    n125 = control-ref of="Tab Body"() -> (w298:refnum<vi>)
                    n126 = call "Tabs - Page Visibility.vi"("Matching Tab#"=w296, "PageLabel"=string[] ["WIN8", "WIN4", "WIN1", "Admin", "Config"], "[TabUserAccess]"="[TabUserAccess]", "TabControl in"=w298) -> ()  [unwired: 7 in, 1 out]
                  }
                }
                n127 = for {
                  tunnel: w155 -> [w222] mode=indexing
                  tunnel: w154 -> [w218]
                  tunnel: w153 -> [w217]
                  tunnel: [w216] -> w151
                  n128 = property class="Page"(reference=w222, error in=w218) -> (reference out=w220:refnum<vi>, error out=w219:errorcluster, "PageLabel"=w221:string)
                  n129 = case shown="\"WIN1\"" w221 {
                    tunnel: w220 -> [_ w229 w235 w241 w247 w253]
                    tunnel: w219 -> [w223 w228 w234 w240 w246 w252]
                    tunnel: w217 -> [_ w227 w233 w239 w245 w251]
                    tunnel: [w223 w224 w230 w236 w242 w248] -> w216
                    frame "False", Default {
                    }
                    frame "WIN8" {
                      n130 = Index Array(array=w227, index=0) -> (element=w225:string)
                      n131 = property class="Page"(reference=w229, error in=w228, "TabCaption"=w225) -> (error out=w224:errorcluster)  [unwired: 1 out]
                    }
                    frame "WIN4" {
                      n132 = Index Array(array=w233, index=1) -> (element=w231:string)
                      n133 = property class="Page"(reference=w235, error in=w234, "TabCaption"=w231) -> (error out=w230:errorcluster)  [unwired: 1 out]
                    }
                    frame "WIN1" {
                      n134 = Index Array(array=w239, index=2) -> (element=w237:string)
                      n135 = property class="Page"(reference=w241, error in=w240, "TabCaption"=w237) -> (error out=w236:errorcluster)  [unwired: 1 out]
                    }
                    frame "Admin" {
                      n136 = Index Array(array=w245, index=11) -> (element=w243:string)
                      n137 = property class="Page"(reference=w247, error in=w246, "TabCaption"=w243) -> (error out=w242:errorcluster)  [unwired: 1 out]
                    }
                    frame "Config" {
                      n138 = Index Array(array=w251, index=12) -> (element=w249:string)
                      n139 = property class="Page"(reference=w253, error in=w252, "TabCaption"=w249) -> (error out=w248:errorcluster)  [unwired: 1 out]
                    }
                  }
                }
                n140 = call <vilib>:"Application Directory.vi"() -> ("Application Directory"=w179:path)
                n141 = Build Path(base path=w179, name or relative path="CMSClient.ini" ("ini Name")) -> (appended path=w176:path)
                n142 = call "DB - [Config].[Parameter].vi"("Application"="CMS", "[PlantId]"=w162, "[ParameterId] Values"=string[] ["DisplayDurationInMin"]) -> ("2D data"=w149:string[][])  [unwired: 6 in, 2 out]
                n143 = call <vilib>:"Open Config Data.vi"("create file if necessary (T)"=FALSE, "configuration file path"=w176) -> ("error out"=w174:errorcluster, "refnum"=w175:T25)  [unwired: 7 in, 1 out]
                n144 = for {
                  tunnel: w149 -> [w211] mode=indexing
                  n145 = Index Array(array=w211) -> (element #1=w210:string, element #2=w209:string)  [unwired: 2 in]
                  n146 = case shown="\"DisplayDurationInMin\"" w210 {
                    tunnel: w209 -> [_ w212]
                    frame "False", Default {
                    }
                    frame "DisplayDurationInMin" {
                      n147 = Decimal String To Number(string=w212) -> (number=w215:i32)  [unwired: 2 in, 1 out]
                      n148 = Max & Min(x=w215, y=10) -> (max(x,y)=→"DisplayDurationInMin":i32)  [unwired: 1 out]
                    }
                  }
                }
                n149 = call-poly <vilib>:"Write Key.vi"("write raw string? (F)"=w170, "section"=w169, "error in (no error)"=w174, "value"=w171, "key"="LogoFile", "refnum"=w175) -> ("error out"=w172:errorcluster, "refnum out"=w173:T25)  [unwired: 3 in, 1 out]
                n150 = call-poly <vilib>:"Write Key.vi"("write raw string? (F)"=w170, "section"=w169, "error in (no error)"=w172, "value"=w167, "key"="Software Solution Name", "refnum"=w173) -> ("error out"=w166:errorcluster, "refnum out"=w165:T25)  [unwired: 3 in, 1 out]
                n151 = call <vilib>:"Close Config Data.vi"("error in (no error)"=w166, "refnum"=w165) -> ("error out"=w164:errorcluster)  [unwired: 8 in, 1 out]
                n152 = Close Reference(reference=w152, error in (no error)=w151) -> (error out=w150:errorcluster)
                n153 = local write "ini File"(w164) -> ()
                n154 = local write "Property Node"(w150) -> ()
                n155 = flat-sequence "CMS only" {
                  tunnel: w206 -> [_]
                  tunnel: [errorcluster {"status"=FALSE, "code"=0, "source"=""} ("error constant")] -> _
                  frame #0 {
                    w271 = string[] ["WIN8", "WIN4", "WIN1"] ("PageLabel")
                    # "Only Show if Exist in WindowView"
                    n156 = global read "Global CMS.vi" "Logon"() -> (w277:T7)
                    n157 = Unbundle By Name(w277) -> ("PlantID"=w276:string, "StationID"=w267:string)
                    "Station" <- w267
                    n158 = Bundle("PlantID"=w276, "StationID"=w267) -> (w280:cluster{"PlantID":string, "StationID":string})  [unwired: 1 in]
                    n159 = call "DB - [CMS].[Config].[WindowView].vi"("DB - CMS Config View"=DB_-_CMS_Config_WindowView."SELECT [Config].[View]", "[PlantId],[StationId]"=w280) -> ("data"=w275:string[][])  [unwired: 11 in, 2 out]
                    "WindowView (ORDERed by DB)" <- w275
                    n160 = Index Array(array=w275, index (col)=0 ("disabled index (col)")) -> (element=w273:string[])  [unwired: 1 in]
                    n161 = for {
                      tunnel: w271 -> [w291] mode=indexing
                      tunnel: w273 -> [w292]
                      tunnel: [w289] -> w270 mode=indexing
                      tunnel: [w288] -> w269 mode=indexing
                      i -> [w288]
                      n162 = Search 1D Array(1D array=w292, element=w291) -> (index of element=w290:i32)  [unwired: 1 in]
                      n163 = Greater Or Equal To 0?(x=w290) -> (x >= 0?=w289:bool)
                    }
                    n164 = control-ref of="Tab Body"() -> (w272:refnum<vi>)
                    n165 = disable-structure shown="Enabled" {
                      disable-tunnel: w272 -> [w287 _]
                      disable-tunnel: w271 -> [w286 _]
                      disable-tunnel: w270 -> [w285 _]
                      disable-tunnel: w269 -> [w284 _]
                      frame Enabled {
                        n166 = call "Tabs - Page Visibility.vi"("Matching Tab#"=w284, "PageLabel"=w286, "[TabUserAccess]"=w285, "TabControl in"=w287) -> ()  [unwired: 7 in, 1 out]
                      }
                      frame Disabled {
                      }
                    }
                    n167 = Index Array(array=w275, index (row)=0 ("disabled index (row)"), index (col)=0 ("disabled index (col)")) -> (element=w279:string)
                    n168 = case shown="\"WIN8\", Default" w279 {
                      tunnel: [CMS_Windows_Tab."WIN1" ("Tab Body") CMS_Windows_Tab."WIN4" ("Tab Body") CMS_Windows_Tab."WIN8" ("Tab Body")] -> w278
                      frame "WIN1" {
                      }
                      frame "WIN4" {
                      }
                      frame "WIN8", Default {
                      }
                    }
                    n169 = local write "Tab Body"(w278) -> ()
                  }
                }
              }
            }
          }
        }
      }
      frame "RUNNING Process" {
        n170 = while {
          tunnel: w302 -> [_]
          tunnel: w301 -> [w311]
          tunnel: [w310] -> w300
          i -> [w328]
          stop <- w313 stop-if-true
          w309 = Enum_-_CMS_State."READY TO START"  # CMS Main Process
          n171 = local read "Skip WIN Timer"() -> (w306:bool)
          n172 = local read "Skip TAB Timer"() -> (w305:bool)
          n173 = Equal To 0?(x=w328) -> (x = 0?=w324:bool)
          n174 = local read "[ToggleTabInterval]"() -> (w322:dbl)
          n175 = local read "[ToggleWinInterval]"() -> (w321:dbl)
          n176 = call "Elapsed Time"("Time Target (s)"=w321, "Reset"=w306) -> ("Elapsed Time (s)"=w327:dbl, "Time has Elapsed"=w323:bool)  [unwired: 10 in, 6 out]
          n177 = local read "Tab Body"() -> (w320:T1)
          n178 = call "Elapsed Time2"("Time Target (s)"=w322, "Reset"=w305) -> ("Elapsed Time (s)"=w325:dbl, "Time has Elapsed"=w304:bool)  [unwired: 10 in, 6 out]
          n179 = case shown="\"WIN8\"..\"WIN1\"" w320 {
            tunnel: [FALSE TRUE] -> w318
            frame Default {
            }
            frame "WIN8".."WIN1" {
              # "Allow Update of WINxx"
            }
          }
          n180 = local read "Reset [TabId] Index"() -> (w316:bool)
          n181 = case shown="True" w305 {
            tunnel: w304 -> [w331 _]
            tunnel: [w331 w332] -> w303
            frame False {
            }
            frame True {
              w332 = TRUE  # Time has Elapsed
              # "Simulate Time has Elapsed\nToggle Back"
              n182 = local write "Skip TAB Timer"(FALSE ("Skip TAB Timer")) -> ()
            }
          }
          n183 = Subtract(x=w322, y=w325) -> (x-y=→"[ToggleTabInterval] Timer":dbl)
          n184 = Subtract(x=w321, y=w327) -> (x-y=→"[ToggleWinInterval] Timer":dbl)
          n185 = case shown="True" w306 {
            frame False {
            }
            frame True {
              # "Toggle Back is now done later"
              n186 = disable-structure shown="Disabled" {
                frame Disabled {
                  n187 = local write "Skip WIN Timer"(FALSE ("Skip Timer")) -> ()
                }
                frame Enabled {
                }
              }
            }
          }
          n188 = Wait Until Next ms Multiple(millisecond multiple=u32 100) -> ()  [unwired: 1 out]
          n189 = Format Date/Time String(time format string (%c)="%b %d, %Y  %H:%M:%S") -> (date/time string=w307:string)  [unwired: 2 in]
          n190 = local write "Date Time"(w307) -> ()
          n191 = Compound Arithmetic op=OR "OR"(w306, w303, w323, w324, w316) -> (w319:bool)
          n192 = And(x=w319, y=w318) -> (x .and. y?=w317:bool)
          n193 = case shown="True" w317 {
            tunnel: w303 -> [_ w363]
            frame False {
            }
            frame True {
              w351 = 60  # sec
              w355 = 2  # SYSDATETIME()
              w356 = 1  # [LastUpdatedCmsTime]
              w357 = 0  # [IsActive]
              w408 = 0  # # of Rows
              # "If Empty may need to hide the WINDOWxx"
              # "1 hour"
              # "[ToggleTabInterval] OR [ToggleWinInterval] Time expired OR i=0 OR Skip Timer \nAND Tab Body = WINx"
              n194 = local read "WindowView (ORDERed by DB)"() -> (w405:string[][])
              n195 = local read "Reset [TabId] Index"() -> (w362:bool)
              n196 = local read "[ToggleTab] Override"() -> (w368:bool)
              n197 = local read "[ToggleTab]"() -> (w369:bool)
              n198 = Array Size(array=w405) -> (size(s)=w410:i32[])
              n199 = Index Array(array=w410, index=w408) -> (element=w409:i32)
              n200 = Compound Arithmetic op=AND "AND"(invert w368, w369, w363) -> (w367:bool)
              n201 = feedback #1(0) -> (w407:i32)
              n202 = case shown="True" w367 {
                tunnel: w407 -> [w578 w580]
                tunnel: [w578 w579] -> w366
                frame False {
                }
                frame True {
                  n203 = Increment(x=w580) -> (x+1=w579:i32)
                }
              }
              n204 = case shown="True" w362 {
                tunnel: w366 -> [w416 _]
                tunnel: [w416 w418] -> w365
                tunnel: [w415 TRUE] -> w364
                tunnel: w363 -> [w415 _]
                frame False {
                }
                frame True {
                  # "Reset [TabId] to current Tab\nReset Window to Window01"
                  n205 = local read "New [TabId] Index"() -> (w418:i32)
                  n206 = local write "Reset [TabId] Index"(FALSE ("Reset [TabId] Index")) -> ()
                }
              }
              "[TabId] Index" <- w365
              n207 = Quotient & Remainder(x=w365, y=w409) -> (x-y*floor(x/y)=w404:i32)  [unwired: 1 out]
              n208 = Index Array(array=w405, index (row)=w404) -> (element=w385:string[])  [unwired: 1 in]
              "Current WindowView" <- w385
              n209 = feedback-in #1(w365) -> ()
              n210 = Index Array(array=w385, index #1=DB_-_Config_WindowView_Enum."w.[TabId]", index #3=DB_-_Config_WindowView_Enum."w.[ToggleTabInterval]", index #4=DB_-_Config_WindowView_Enum."w.[ToggleWinInterval]", index #5=DB_-_Config_WindowView_Enum."v.[ToggleTab]") -> (element #1=w400:string, element #3=w384:string, element #4=w383:string, element #5=w382:string)  [unwired: 1 in, 1 out]
              "Current [TabId]" <- w400
              n211 = To Upper Case(1:w400) -> (0:w376:string)
              n212 = call "DB - Convert BIT Type.vi"("BIT Type (eg Inactive)"=w382) -> ("Boolean"=w370:bool)  [unwired: 2 in, 2 out]
              n213 = local read "Min [ToggleWinInterval]"() -> (w386:i32)
              n214 = local read "Min [ToggleTabInterval]"() -> (w387:i32)
              n215 = case shown="\"WIN8\"" w376 {
                tunnel: [1 4 8 16] -> _
                tunnel: [CMS_Windows_Tab."WIN1" ("Tab Body") CMS_Windows_Tab."WIN4" ("Tab Body") CMS_Windows_Tab."WIN8" ("Tab Body") CMS_Windows_Tab."WIN8" ("Tab Body")] -> w399
                frame "WIN1", Default {
                }
                frame "WIN4" {
                }
                frame "WIN8" {
                }
                frame "WIN16" {
                }
              }
              n216 = local write "[ToggleTab]"(w370) -> ()
              n217 = Decimal String To Number(string=w384) -> (number=w390:i32)  [unwired: 2 in, 1 out]
              n218 = Decimal String To Number(string=w383) -> (number=w388:i32)  [unwired: 2 in, 1 out]
              n219 = Max & Min "At Least 30seconds"(x=w390, y=w387) -> (max(x,y)=w391:i32)  [unwired: 1 out]
              n220 = Max & Min "At Least 2seconds"(x=w388, y=w386) -> (max(x,y)=w389:i32)  [unwired: 1 out]
              n221 = case shown="True" w367 {
                tunnel: w399 -> [_ w420]
                frame False {
                }
                frame True {
                  n222 = local write "Tab Body"(w420) -> ()
                }
              }
              n223 = local write "[ToggleTabInterval]"(w391) -> ()
              n224 = local write "[ToggleWinInterval]"(w389) -> ()
              n225 = feedback #2(0) -> (w403:i32)
              n226 = Select(t=0, s=w364, f=w403) -> (s? t:f=w401:i32)
              n227 = while {
                tunnel: w385 -> [w577]
                tunnel: DB_-_Config_WindowView_Enum."w.[Window01]" -> [w574]
                shift-right: [w566] -> w398
                shift-left: w401 -> [w572]
                tunnel: 24 -> [w568]
                tunnel: [w567] -> w360
                tunnel: [w567] -> w342 mode=indexing if=w565
                tunnel: [w566] -> _ mode=indexing if=w565
                i -> [w570]
                stop <- w576 stop-if-true
                # "If it goes more than 1 round there is \nan error!"
                n228 = Quotient & Remainder(x=w572, y=w568) -> (x-y*floor(x/y)=w571:i32)  [unwired: 1 out]
                n229 = Add(x=w574, y=w571) -> (x+y=w573:i32)
                n230 = Equal?(x=w568, y=w570) -> (x = y?=w569:bool)
                n231 = Index Array(array=w577, index=w573) -> (element=w567:string)
                "[WINDOWxx]" <- w567
                n232 = Increment(x=w571) -> (x+1=w566:i32)
                n233 = Empty String/Path?(string/path=w567) -> (empty?=w565:bool)
                n234 = Not "NotEmptyString"(x=w565) -> (.not. x?=w575:bool)
                n235 = Compound Arithmetic op=OR(w575, w569) -> (w576:bool)
              }
              "Empty [WINDOWxx]" <- w342
              n236 = feedback-in #2(w398) -> ()
              n237 = Decrement(x=w398) -> (x-1=w392:i32)
              n238 = local read "Stay in [WINDOWxx]"() -> (w361:bool)
              n239 = case shown="\"WIN8\"" w376 {
                tunnel: [w539 w545 w553] -> w397
                tunnel: w392 -> [_ w547 w554]
                tunnel: [w540 w544 w549] -> w372
                tunnel: [FALSE w541 w550] -> w373
                frame "WIN1", Default {
                  n240 = control-ref of="Cluster0 WIN1"() -> (w539:refnum<vi>)
                  n241 = Build Array(w539) -> (w540:refnum<vi>[])
                }
                frame "WIN4" {
                  n242 = local read "WIN4 Array"() -> (w544:refnum<vi>[])
                  n243 = local read "WIN4 IQ"() -> (w542:i32)
                  n244 = Quotient & Remainder(x=w547, y=4) -> (x-y*floor(x/y)=w546:i32, floor(x/y)=w543:i32)
                  "WIN4 IQ" <- w543
                  n245 = Not Equal?(x=w543, y=w542) -> (x != y?=w541:bool)
                  n246 = Index Array(array=w544, index=w546) -> (element=w545:refnum<vi>)
                }
                frame "WIN8" {
                  n247 = local read "WIN8 Array"() -> (w549:refnum<vi>[])
                  n248 = local read "WIN8 IQ"() -> (w551:i32)
                  n249 = Quotient & Remainder(x=w554, y=8) -> (x-y*floor(x/y)=w556:i32, floor(x/y)=w552:i32)
                  "WIN8 IQ" <- w552
                  n250 = Not Equal?(x=w552, y=w551) -> (x != y?=w550:bool)
                  n251 = Index Array(array=w549, index=w556) -> (element=w553:refnum<vi>)
                }
              }
              n252 = local read "[WINDOWxx] Stay"() -> (w358:string)
              n253 = Select(t=w358, s=w361, f=w360) -> (s? t:f=w359:string)
              n254 = xnode "Match Regular Expression"("input string"=w359, "regular expression"="\\.") -> ("before match"=w394:string, "after match"=w393:string)  [unwired: 4 in, 3 out]
              n255 = Bundle(cluster=cluster{"PlantID":string, "SystemID":string} {"PlantID"="", "SystemID"=""}, "PlantID"=w394, "SystemID"=w393) -> (w411:cluster{"PlantID":string, "SystemID":string})
              n256 = local read "DisplayDurationInMin"() -> (w337:i32)
              n257 = call "DB - [CMS].[Execute].[ActiveProcess].vi"("Application"="CMS", "[PlantId],[SystemId]"=w411, "DB - CMS Execute ActiveProcess"=DB_-_CMS_Execute_Active_Process."Check [IsActive]" ("DB - Execute ActiveProcess")) -> ("data"=w340:string[], "SUMMARY"=w412:errorcluster)  [unwired: 13 in, 2 out]
              n258 = Get Date/Time In Seconds() -> (seconds since 1Jan1904=w346:timestamp)
              n259 = Index Array(array=w340, index #1=w357, index #2=w356, index #3=w355) -> (element #1=w413:string, element #2=w353:string, element #3=w354:string)
              n260 = case shown="True" w373 {
                tunnel: w372 -> [w421 w422]
                tunnel: [w421 w422] -> w371
                frame False {
                  # "\"Same Page\""
                }
                frame True {
                  # "Refresh (\"Next Page\")"
                  n261 = for {
                    tunnel: w422 -> [w423] mode=indexing
                    n262 = invoke class="Clust (strict)" method="Reinit To Default"(reference=w423) -> ()  [unwired: 2 in, 3 out]
                  }
                }
              }
              n263 = Empty Array?(array=w340) -> (empty?=w338:bool)
              n264 = call "String - Convert Str (YYYY-mm-dd HHcMMcSS) to TimeStamp.vi"("YYYY-mm-dd HH:MM:SS (String)"=w354) -> ("time stamp"=w347:timestamp)  [unwired: 9 in, 1 out]
              n265 = call "String - Convert Str (YYYY-mm-dd HHcMMcSS) to TimeStamp.vi"("YYYY-mm-dd HH:MM:SS (String)"=w353) -> ("time stamp"=w345:timestamp)  [unwired: 9 in, 1 out]
              n266 = call "DB - Convert BIT Type.vi"("BIT Type (eg Inactive)"=w413) -> ("Boolean"=w348:bool)  [unwired: 2 in, 2 out]
              n267 = Multiply(x=w337, y=w351) -> (x*y=w350:i32)
              n268 = Subtract(x=w347, y=w345) -> (x-y=w352:dbl)
              n269 = Subtract(x=w347, y=w346) -> (x-y=w344:dbl)
              "Time Offset" <- w344
              n270 = Less?(x=w352, y=w350) -> (x < y?=w349:bool)
              n271 = Or(x=w348, y=w349) -> (x .or. y?=w339:bool)
              n272 = Add(x=w345, y=w344) -> (x+y=w343:timestamp)
              n273 = case shown="False" w339 {
                tunnel: w411 -> [w593 w1017]
                tunnel: w412 -> [w598 _]
                tunnel: w397 -> [w592 w1016]
                tunnel: w371 -> [w591 w1015]
                tunnel: w376 -> [w590 w1014]
                tunnel: w343 -> [w585 _]
                tunnel: w338 -> [w583 _]
                frame True {
                  w586 = "%Y-%m-%d %H:%M"  # Last Updated On Format
                  w588 = T23[] [enum."[TransactionNo]", enum."[TransactionRunNo]", enum."[RecordedMinutes]", enum."[HoldTimeRemaining]", enum."[HoldProgressColor]", enum."[ProcessColor]", enum."[OverallColor]", enum."[ControllerStatus]", enum."[IsControllerOnline]", enum."[FurnaceControlStatus]", enum."[FurnaceControlColor]"] items=["[IsActive]", "[TransactionNo]", "[TransactionRunNo]", "[SequenceStatus]", "[StartRecordTime]", "[EndRecordTime]", "[StartHoldTime]", "[EndHoldTime]", "[Message1]", "[Message2]", "[HoldTimeRemaining]", "[HoldTimePercentage]", "[HoldProgressColor]", "[OrderNumbers]", "[CurrentTemp]", "[UnitOfTemperature]", "[IsAppClientLive]", "[RawDataFile]", "[RecordedMinutes]", "[FurnaceControlStatus]", "[FurnaceControlColor]", "[ControllerStatus]", "[ControllerColor]", "[IsControllerOnline]", "[ProcessColor]", "[OverallColor]", "[LastUpdatedOn]", "[LastUpdatedCmsTime]", "[Inactive]"] ("[Execute].[ActiveProcess]\n2014-10-14 14:58")
                  w589 = T23[] [enum."[CurrentTemp]", enum."[UnitOfTemperature]", enum."[SequenceStatus]", enum."[StartRecordTime]", enum."[EndRecordTime]", enum."[StartHoldTime]", enum."[EndHoldTime]", enum."[HoldTimePercentage]", enum."[ControllerColor]", enum."[LastUpdatedOn]", enum."[Message1]"] items=["[IsActive]", "[TransactionNo]", "[TransactionRunNo]", "[SequenceStatus]", "[StartRecordTime]", "[EndRecordTime]", "[StartHoldTime]", "[EndHoldTime]", "[Message1]", "[Message2]", "[HoldTimeRemaining]", "[HoldTimePercentage]", "[HoldProgressColor]", "[OrderNumbers]", "[CurrentTemp]", "[UnitOfTemperature]", "[IsAppClientLive]", "[RawDataFile]", "[RecordedMinutes]", "[FurnaceControlStatus]", "[FurnaceControlColor]", "[ControllerStatus]", "[ControllerColor]", "[IsControllerOnline]", "[ProcessColor]", "[OverallColor]", "[LastUpdatedOn]", "[LastUpdatedCmsTime]", "[Inactive]"] ("[Execute].[ActiveProcess]\n2014-10-14 14:58")
                  # "Reset Skip Timer"
                  # "Not used for WIN1"
                  # "IsActive OR <60min"
                  n274 = local write "Skip WIN Timer"(FALSE ("Skip Timer")) -> ()
                  n275 = local write "Skip Timer Count"(0 ("Skip Timer Count")) -> ()
                  n276 = property class="Clust (strict)"(reference=w592) -> ("Controls[]"=w599:refnum<vi>[])  [unwired: 1 in, 2 out]
                  n277 = Build Array (concatenate)(w589, w588) -> (w587:T23[])
                  n278 = for {
                    tunnel: w587 -> [w1013] mode=indexing
                    tunnel: [w1012] -> w596 mode=indexing
                    n279 = Format Into String(w1013) -> (resulting string=w1012:string)  [unwired: 3 in, 1 out]
                  }
                  n280 = call "DB - [CMS].[Execute].[ActiveProcess].vi"("Application"="CMS", "[PlantId],[SystemId]"=w593, "error in (no error)"=w598, "DB - CMS Execute ActiveProcess"=DB_-_CMS_Execute_Active_Process."SELECT [Execute].[ActiveProcess]" ("DB - Execute ActiveProcess"), "[Execute].[ActiveProcess]\n2014-10-14 14:58"=w587) -> ("data"=w597:string[], "SUMMARY"=w594:errorcluster)  [unwired: 11 in, 2 out]
                  "DB" <- w594
                  n281 = case shown="\"WIN4\", \"WIN8\"" w590 {
                    tunnel: w599 -> [_ w714]
                    tunnel: w597 -> [w630 w713]
                    tunnel: w596 -> [w631 w712]
                    tunnel: w594 -> [w642 w711]
                    tunnel: w593 -> [w606 w710]
                    tunnel: w591 -> [_ w709]
                    tunnel: w586 -> [w603 w708]
                    tunnel: w585 -> [_ w706]
                    tunnel: w583 -> [_ w705]
                    frame "WIN1", Default {
                      w611 = 60.0  # 60sec
                      w615 = 60.0  # 60sec
                      w632 = T23[] [enum."[StartRecordTime]", enum."[LastUpdatedOn]"] items=["[IsActive]", "[TransactionNo]", "[TransactionRunNo]", "[SequenceStatus]", "[StartRecordTime]", "[EndRecordTime]", "[StartHoldTime]", "[EndHoldTime]", "[Message1]", "[Message2]", "[HoldTimeRemaining]", "[HoldTimePercentage]", "[HoldProgressColor]", "[OrderNumbers]", "[CurrentTemp]", "[UnitOfTemperature]", "[IsAppClientLive]", "[RawDataFile]", "[RecordedMinutes]", "[FurnaceControlStatus]", "[FurnaceControlColor]", "[ControllerStatus]", "[ControllerColor]", "[IsControllerOnline]", "[ProcessColor]", "[OverallColor]", "[LastUpdatedOn]", "[LastUpdatedCmsTime]", "[Inactive]"]
                      w651 = T23[] [enum."[SequenceStatus]", enum."[ControllerStatus]", enum."[ControllerColor]", enum."[IsControllerOnline]", enum."[FurnaceControlStatus]", enum."[FurnaceControlColor]"] items=["[IsActive]", "[TransactionNo]", "[TransactionRunNo]", "[SequenceStatus]", "[StartRecordTime]", "[EndRecordTime]", "[StartHoldTime]", "[EndHoldTime]", "[Message1]", "[Message2]", "[HoldTimeRemaining]", "[HoldTimePercentage]", "[HoldProgressColor]", "[OrderNumbers]", "[CurrentTemp]", "[UnitOfTemperature]", "[IsAppClientLive]", "[RawDataFile]", "[RecordedMinutes]", "[FurnaceControlStatus]", "[FurnaceControlColor]", "[ControllerStatus]", "[ControllerColor]", "[IsControllerOnline]", "[ProcessColor]", "[OverallColor]", "[LastUpdatedOn]", "[LastUpdatedCmsTime]", "[Inactive]"]
                      w661 = T23[] [enum."[HoldTimePercentage]", enum."[HoldProgressColor]", enum."[ProcessColor]", enum."[OverallColor]"] items=["[IsActive]", "[TransactionNo]", "[TransactionRunNo]", "[SequenceStatus]", "[StartRecordTime]", "[EndRecordTime]", "[StartHoldTime]", "[EndHoldTime]", "[Message1]", "[Message2]", "[HoldTimeRemaining]", "[HoldTimePercentage]", "[HoldProgressColor]", "[OrderNumbers]", "[CurrentTemp]", "[UnitOfTemperature]", "[IsAppClientLive]", "[RawDataFile]", "[RecordedMinutes]", "[FurnaceControlStatus]", "[FurnaceControlColor]", "[ControllerStatus]", "[ControllerColor]", "[IsControllerOnline]", "[ProcessColor]", "[OverallColor]", "[LastUpdatedOn]", "[LastUpdatedCmsTime]", "[Inactive]"]
                      w662 = T23[] [enum."[TransactionNo]", enum."[TransactionRunNo]", enum."[RecordedMinutes]", enum."[HoldTimeRemaining]", enum."[CurrentTemp]", enum."[UnitOfTemperature]"] items=["[IsActive]", "[TransactionNo]", "[TransactionRunNo]", "[SequenceStatus]", "[StartRecordTime]", "[EndRecordTime]", "[StartHoldTime]", "[EndHoldTime]", "[Message1]", "[Message2]", "[HoldTimeRemaining]", "[HoldTimePercentage]", "[HoldProgressColor]", "[OrderNumbers]", "[CurrentTemp]", "[UnitOfTemperature]", "[IsAppClientLive]", "[RawDataFile]", "[RecordedMinutes]", "[FurnaceControlStatus]", "[FurnaceControlColor]", "[ControllerStatus]", "[ControllerColor]", "[IsControllerOnline]", "[ProcessColor]", "[OverallColor]", "[LastUpdatedOn]", "[LastUpdatedCmsTime]", "[Inactive]"]
                      # "Array of up to 4 (Foreground Color, Background Color) pairs, where Foreground Color is the foreground color of the Boolean control and Background Color is the background color of the Boolean control. Color pairs include False, True, True to False, and False to True."
                      n282 = disable-structure shown="Disabled" {
                        frame Disabled {
                          # "4 Signifcant Digits"
                          n283 = Format Value(format string="%#_4") -> ()  [unwired: 2 in, 1 out]
                        }
                        frame Enabled {
                        }
                      }
                      n284 = Unbundle By Name(w606) -> ("SystemID"=→"WIN1 Bay":string)
                      n285 = call "DB - [CMS].[Execute].[ActiveProcess].vi"("Application"="CMS", "[PlantId],[SystemId]"=w606, "error in (no error)"=w642, "DB - CMS Execute ActiveProcess"=DB_-_CMS_Execute_Active_Process."SELECT FILESTREAM" ("DB - Execute ActiveProcess")) -> ("String ([RawDataFile] Filestream)"=w607:string, "SUMMARY"=w643:errorcluster)  [unwired: 12 in, 2 out]
                      n286 = local write "DB"(w643) -> ()
                      n287 = for {
                        tunnel: w662 -> [w702] mode=indexing
                        tunnel: w631 -> [w701]
                        tunnel: w630 -> [w699]
                        tunnel: [w698] -> w672 mode=indexing
                        n288 = Format Into String(w702) -> (resulting string=w703:string)  [unwired: 3 in, 1 out]
                        n289 = Search 1D Array(1D array=w701, element=w703) -> (index of element=w700:i32)  [unwired: 1 in]
                        n290 = Index Array(array=w699, index=w700) -> (element=w698:string)
                      }
                      n291 = for {
                        tunnel: w661 -> [w696] mode=indexing
                        tunnel: w631 -> [w695]
                        tunnel: w630 -> [w693]
                        tunnel: [w692] -> w660 mode=indexing
                        n292 = Format Into String(w696) -> (resulting string=w697:string)  [unwired: 3 in, 1 out]
                        n293 = Search 1D Array(1D array=w695, element=w697) -> (index of element=w694:i32)  [unwired: 1 in]
                        n294 = Index Array(array=w693, index=w694) -> (element=w692:string)
                      }
                      n295 = for {
                        tunnel: w651 -> [w690] mode=indexing
                        tunnel: w631 -> [w689]
                        tunnel: w630 -> [w687]
                        tunnel: [w686] -> w652 mode=indexing
                        n296 = Format Into String(w690) -> (resulting string=w691:string)  [unwired: 3 in, 1 out]
                        n297 = Search 1D Array(1D array=w689, element=w691) -> (index of element=w688:i32)  [unwired: 1 in]
                        n298 = Index Array(array=w687, index=w688) -> (element=w686:string)
                      }
                      n299 = for {
                        tunnel: w632 -> [w684] mode=indexing
                        tunnel: w631 -> [w683]
                        tunnel: w630 -> [w681]
                        tunnel: [w680] -> w629 mode=indexing
                        n300 = Format Into String(w684) -> (resulting string=w685:string)  [unwired: 3 in, 1 out]
                        n301 = Search 1D Array(1D array=w683, element=w685) -> (index of element=w682:i32)  [unwired: 1 in]
                        n302 = Index Array(array=w681, index=w682) -> (element=w680:string)
                      }
                      n303 = Index Array(array=w672) -> (element #1=→"Transaction No (Execute)":string, element #2=→"TransactionRunNo (Execute)":string, element #3=w671:string, element #4=w617:string, element #5=w670:string, element #6=w656:string)  [unwired: 6 in]
                      n304 = Index Array(array=w660) -> (element #1=w659:string, element #2=w658:string, element #3=w657:string, element #4=w653:string)  [unwired: 4 in]
                      n305 = Index Array(array=w652) -> (element #1=→"Sequence Status":string, element #2=→"cRIO Status":string, element #3=w648:string, element #5=→"ET3504 Status":string, element #6=w646:string)  [unwired: 7 in, 2 out]
                      n306 = Index Array(array=w629) -> (element #1=w628:string, element #2=w602:string)  [unwired: 2 in]
                      n307 = call "String - Convert Str (YYYY-mm-dd HHcMMcSS) to TimeStamp.vi"("YYYY-mm-dd HH:MM:SS (String)"=w602) -> ("time stamp"=w604:timestamp)  [unwired: 9 in, 1 out]
                      n308 = Format Date/Time String(time format string (%c)=w603, seconds (now)=w604) -> (date/time string=→"Last Updated On":string)  [unwired: 1 in]
                      n309 = Fract/Exp String To Number(string=w671) -> (number=w613:dbl)  [unwired: 3 in, 1 out]
                      n310 = Fract/Exp String To Number(string=w617) -> (number=w616:dbl)  [unwired: 3 in, 1 out]
                      n311 = Fract/Exp String To Number(string=w670) -> (number=w669:dbl)  [unwired: 3 in, 1 out]
                      n312 = call "String - Convert Str (YYYY-mm-dd HHcMMcSS) to TimeStamp.vi"("YYYY-mm-dd HH:MM:SS (String)"=w628) -> ("time stamp"=w627:timestamp)  [unwired: 9 in, 1 out]
                      n313 = call "Chart - Load History.vi"("time stamp"=w627, "Filestream"=w607, "Load From File"=FALSE) -> ("Error Out"=w639:errorcluster, "Plot Names"=w610:string[], "History"=w641:dynamicdata[])  [unwired: 3 in, 3 out]
                      n314 = property on="Chart" class="WFChart (strict)"(error in=w639, "History Data"=w641) -> (error out=w609:errorcluster)  [unwired: 1 in, 1 out]
                      n315 = Fract/Exp String To Number(string=w659) -> (number=w626:dbl)  [unwired: 3 in, 1 out]
                      "% Hold. Time Completed" <- w626
                      n316 = Decimal String To Number(string=w658) -> (number=w665:i32)  [unwired: 2 in, 1 out]
                      n317 = Decimal String To Number(string=w657) -> (number=w663:i32)  [unwired: 2 in, 1 out]
                      n318 = Decimal String To Number(string=w653) -> (number=w655:i32)  [unwired: 2 in, 1 out]
                      n319 = Decimal String To Number(string=w648) -> (number=w673:i32)  [unwired: 2 in, 1 out]
                      n320 = Decimal String To Number(string=w646) -> (number=w647:i32)  [unwired: 2 in, 1 out]
                      n321 = Multiply(x=w615, y=w616) -> (x*y=w614:dbl)
                      n322 = Multiply(x=w611, y=w613) -> (x*y=w612:dbl)
                      n323 = Bundle(w665, w665) -> (w620:cluster{i32, i32})  [unwired: 1 in]
                      n324 = property on="cRIO Status" class="Str"("Text.BG Color"=w673) -> (error out=w635:errorcluster)  [unwired: 2 in, 1 out]
                      n325 = Bundle By Name(cluster=T4 {"Recording Duration"=0.0, "Remaining Hold Time"=0.0, "Current Temp"=0.0, "Key Values Temperature Units"=""} ("Key Values"), "Recording Duration"=w612, "Remaining Hold Time"=w614, "Current Temp"=w669, "Key Values Temperature Units"=w656) -> (→"Key Values":T4)
                      n326 = property on="ET3504 Status" class="Str"("Text.BG Color"=w647) -> (error out=w634:errorcluster)  [unwired: 2 in, 1 out]
                      n327 = Bundle(w663, w663) -> (w619:cluster{i32, i32})  [unwired: 1 in]
                      n328 = Bundle(w655, w655) -> (w618:cluster{i32, i32})  [unwired: 1 in]
                      n329 = Build Array(w620, w620) -> (w666:cluster{i32, i32}[])
                      n330 = Build Array(w619, w619) -> (w664:cluster{i32, i32}[])
                      n331 = Build Array(w618, w618) -> (w654:cluster{i32, i32}[])
                      n332 = property on="Process Completed" class="Bool (strict)"("Colors [4]"=w664) -> (error out=w637:errorcluster)  [unwired: 2 in, 1 out]
                      n333 = property on="Overall Status" class="Bool (strict)"("Colors [4]"=w654) -> (error out=w636:errorcluster)  [unwired: 2 in, 1 out]
                      n334 = property on="Hold Time Completed" class="Bool (strict)"("Colors [4]"=w666) -> (error out=w638:errorcluster)  [unwired: 2 in, 1 out]
                      n335 = for {
                        tunnel: w610 -> [w678] mode=indexing
                        tunnel: w609 -> [w677]
                        tunnel: [w676] -> w608
                        i -> [w679]
                        n336 = property on="Chart" class="WFChart (strict)"(error in=w677, "Active Plot"=w679, "Plot.Plot Name"=w678) -> (error out=w676:errorcluster)  [unwired: 1 in, 1 out]
                      }
                      "Load History" <- w608
                      n337 = Merge Errors(w638, w637, w636, w635, w634) -> (→"Property Node":errorcluster)
                      n338 = Greater Or Equal?(x=w626, y=1.0) -> (x >= y?=w623:bool)
                      n339 = Select(t=u32 6618880, s=w623, f=u32 16777216) -> (s? t:f=w624:u32)
                      n340 = property on="% Hold. Time Completed" class="Slide (strict)"("Fill Color"=w624) -> ()  [unwired: 2 in, 2 out]
                    }
                    frame "WIN4", "WIN8" {
                      n341 = disable-structure shown="Disabled" {
                        disable-tunnel: [w719 _] -> w707
                        disable-tunnel: w705 -> [w716 _]
                        frame Disabled {
                          n342 = Format Into String(DB_-_[Execute].[ActiveProcess]_Enum."[ControllerStatus]" ("[Execute].[ActiveProcess]\n2014-10-14 14:58")) -> (resulting string=w721:string)  [unwired: 3 in, 1 out]
                          n343 = To Upper Case(1:w721) -> (0:w722:string)
                          n344 = Match Pattern(string=w722, regular expression="OFFLINE") -> (offset past match=w724:i32)  [unwired: 1 in, 3 out]
                          n345 = Greater Or Equal To 0?(x=w724) -> (x >= 0?=w717:bool)
                          n346 = Or(x=w717, y=w716) -> (x .or. y?=w715:bool)
                          n347 = Select(t=u32 16711699, s=w715, f=u32 6618880) -> (s? t:f=w719:u32)
                        }
                        frame Enabled {
                        }
                      }
                      n348 = for {
                        tunnel: w714 -> [w740] mode=indexing
                        tunnel: w713 -> [w737]
                        tunnel: w712 -> [w736]
                        tunnel: w710 -> [w735]
                        tunnel: w711 -> [w734]
                        tunnel: w708 -> [w733]
                        tunnel: w709 -> [w732]
                        tunnel: w707 -> [w728]
                        tunnel: w706 -> [w727]
                        tunnel: w705 -> [w726]
                        i -> [w731]
                        n349 = property class="Ctl"(reference=w740) -> (reference out=w739:refnum<vi>, error out=w729:errorcluster, "Label.Text"=w738:string)  [unwired: 1 in]
                        n350 = case shown="\"Last Updated (Local)\"" w738 {
                          tunnel: w739 -> [w749 w762 w775 w795 w827 w845 w870 w883 w915 w935 w953 w978 w999]
                          tunnel: w737 -> [_ _ w768 w786 w816 w844 w860 w878 w909 _ w948 _ _]
                          tunnel: w736 -> [_ _ w769 w787 w819 w843 w861 w877 w892 _ w949 _ _]
                          tunnel: w735 -> [w748 w760 _ _ _ _ _ _ _ w920 _ w969 _]
                          tunnel: w734 -> [_ _ _ _ _ _ _ _ _ w930 _ _ _]
                          tunnel: w733 -> [_ _ _ w779 w811 _ _ _ _ _ w947 w977 _]
                          tunnel: w732 -> [_ _ _ _ _ _ _ _ _ _ _ _ w997]
                          tunnel: w731 -> [_ _ _ _ _ _ _ _ _ _ _ _ w996]
                          tunnel: [w742 w759 w766 w778 w810 w842 w867 w873 w908 w919 w946 w976 w993] -> w730
                          tunnel: w729 -> [w744 w758 w765 w777 w809 w841 w866 w872 w907 w918 w945 w975 w991]
                          tunnel: w728 -> [_ _ _ _ _ w840 _ _ _ _ _ _ _]
                          tunnel: w727 -> [_ _ _ _ _ _ _ _ _ _ _ w961 _]
                          tunnel: w726 -> [_ w753 _ _ _ _ _ _ w896 _ _ _ _]
                          frame "[PlantId.SystemId]" {
                            w750 = refnum<vi> refnum  # String
                            n351 = Unbundle By Name(w748) -> ("PlantID"=w747:string, "SystemID"=w745:string)
                            n352 = To More Specific Class(target class=w750, reference=w749, error in=w744) -> (specific class reference=w751:refnum<vi>, error out=w743:errorcluster)
                            n353 = Concatenate Strings(w747, "." ("string"), w745) -> (w741:string)
                            n354 = property class="Str"(reference=w751, error in=w743, "Value"=w741) -> (error out=w742:errorcluster)  [unwired: 1 out]
                          }
                          frame "Bay", Default {
                            w763 = refnum<vi> refnum  # String
                            n355 = Unbundle By Name(w760) -> ("SystemID"=w754:string)
                            n356 = To More Specific Class(target class=w763, reference=w762, error in=w758) -> (specific class reference=w761:refnum<vi>, error out=w757:errorcluster)
                            n357 = Concatenate Strings(w754, " (Offline)" ("string")) -> (w755:string)
                            n358 = Select(t=w755, s=w753, f=w754) -> (s? t:f=w752:string)
                            n359 = property class="Str"(reference=w761, error in=w757, "Text.Text"=w752) -> (error out=w759:errorcluster)  [unwired: 1 out]
                          }
                          frame "Seq Status" {
                            w774 = refnum<vi> refnum  # String
                            n360 = Format Into String(DB_-_[Execute].[ActiveProcess]_Enum."[SequenceStatus]" ("[Execute].[ActiveProcess]\n2014-10-14 14:58")) -> (resulting string=w771:string)  [unwired: 3 in, 1 out]
                            n361 = Search 1D Array(1D array=w769, element=w771) -> (index of element=w770:i32)  [unwired: 1 in]
                            n362 = To More Specific Class(target class=w774, reference=w775, error in=w765) -> (specific class reference=w773:refnum<vi>, error out=w764:errorcluster)
                            n363 = Index Array(array=w768, index=w770) -> (element=w767:string)
                            n364 = property class="Str"(reference=w773, error in=w764, "Text.Text"=w767) -> (error out=w766:errorcluster)  [unwired: 1 out]
                          }
                          frame "Record" {
                            w794 = refnum<vi> refnum  # String
                            n365 = Format Into String(DB_-_[Execute].[ActiveProcess]_Enum."[StartRecordTime]" ("[Execute].[ActiveProcess]\n2014-10-14 14:58")) -> (resulting string=w791:string)  [unwired: 3 in, 1 out]
                            n366 = Format Into String(DB_-_[Execute].[ActiveProcess]_Enum."[EndRecordTime]" ("[Execute].[ActiveProcess]\n2014-10-14 14:58")) -> (resulting string=w788:string)  [unwired: 3 in, 1 out]
                            n367 = Search 1D Array(1D array=w787, element=w791) -> (index of element=w790:i32)  [unwired: 1 in]
                            n368 = Search 1D Array(1D array=w787, element=w788) -> (index of element=w785:i32)  [unwired: 1 in]
                            n369 = To More Specific Class(target class=w794, reference=w795, error in=w777) -> (specific class reference=w793:refnum<vi>, error out=w776:errorcluster)
                            n370 = Index Array(array=w786, index=w790) -> (element=w782:string)
                            n371 = Index Array(array=w786, index=w785) -> (element=w781:string)
                            n372 = case shown="\"True\", Default" w782 {
                              selector: w782 -> [_ w796]
                              tunnel: [_ w800] -> w784
                              tunnel: w779 -> [_ w797]
                              frame "" {
                              }
                              frame "True", Default {
                                n373 = call "String - Convert Str (YYYY-mm-dd HHcMMcSS) to TimeStamp.vi"("YYYY-mm-dd HH:MM:SS (String)"=w796) -> ("time stamp"=w801:timestamp)  [unwired: 9 in, 1 out]
                                n374 = Format Date/Time String(time format string (%c)=w797, seconds (now)=w801) -> (date/time string=w798:string)  [unwired: 1 in]
                                n375 = Concatenate Strings("S: " ("string"), w798) -> (w800:string)
                              }
                            }
                            n376 = case shown="\"True\", Default" w781 {
                              selector: w781 -> [_ w802]
                              tunnel: [_ w804] -> w783
                              tunnel: w779 -> [_ w803]
                              frame "" {
                              }
                              frame "True", Default {
                                n377 = call "String - Convert Str (YYYY-mm-dd HHcMMcSS) to TimeStamp.vi"("YYYY-mm-dd HH:MM:SS (String)"=w802) -> ("time stamp"=w807:timestamp)  [unwired: 9 in, 1 out]
                                n378 = Format Date/Time String(time format string (%c)=w803, seconds (now)=w807) -> (date/time string=w805:string)  [unwired: 1 in]
                                n379 = Concatenate Strings("    E: " ("string"), w805) -> (w804:string)
                              }
                            }
                            n380 = Concatenate Strings(w784, w783) -> (w780:string)
                            n381 = property class="Str"(reference=w793, error in=w776, "Text.Text"=w780) -> (error out=w778:errorcluster)  [unwired: 1 out]
                          }
                          frame "Hold" {
                            w826 = refnum<vi> refnum  # String
                            n382 = Format Into String(DB_-_[Execute].[ActiveProcess]_Enum."[StartHoldTime]" ("[Execute].[ActiveProcess]\n2014-10-14 14:58")) -> (resulting string=w823:string)  [unwired: 3 in, 1 out]
                            n383 = Format Into String(DB_-_[Execute].[ActiveProcess]_Enum."[EndHoldTime]" ("[Execute].[ActiveProcess]\n2014-10-14 14:58")) -> (resulting string=w820:string)  [unwired: 3 in, 1 out]
                            n384 = Search 1D Array(1D array=w819, element=w823) -> (index of element=w822:i32)  [unwired: 1 in]
                            n385 = Search 1D Array(1D array=w819, element=w820) -> (index of element=w821:i32)  [unwired: 1 in]
                            n386 = To More Specific Class(target class=w826, reference=w827, error in=w809) -> (specific class reference=w825:refnum<vi>, error out=w808:errorcluster)
                            n387 = Index Array(array=w816, index=w822) -> (element=w812:string)
                            n388 = Index Array(array=w816, index=w821) -> (element=w813:string)
                            n389 = case shown="\"True\", Default" w812 {
                              selector: w812 -> [_ w828]
                              tunnel: [_ w832] -> w817
                              tunnel: w811 -> [_ w829]
                              frame "" {
                              }
                              frame "True", Default {
                                n390 = call "String - Convert Str (YYYY-mm-dd HHcMMcSS) to TimeStamp.vi"("YYYY-mm-dd HH:MM:SS (String)"=w828) -> ("time stamp"=w833:timestamp)  [unwired: 9 in, 1 out]
                                n391 = Format Date/Time String(time format string (%c)=w829, seconds (now)=w833) -> (date/time string=w830:string)  [unwired: 1 in]
                                n392 = Concatenate Strings("S: " ("string"), w830) -> (w832:string)
                              }
                            }
                            n393 = case shown="\"True\", Default" w813 {
                              selector: w813 -> [_ w834]
                              tunnel: [_ w836] -> w814
                              tunnel: w811 -> [_ w835]
                              frame "" {
                              }
                              frame "True", Default {
                                n394 = call "String - Convert Str (YYYY-mm-dd HHcMMcSS) to TimeStamp.vi"("YYYY-mm-dd HH:MM:SS (String)"=w834) -> ("time stamp"=w839:timestamp)  [unwired: 9 in, 1 out]
                                n395 = Format Date/Time String(time format string (%c)=w835, seconds (now)=w839) -> (date/time string=w837:string)  [unwired: 1 in]
                                n396 = Concatenate Strings("    E: " ("string"), w837) -> (w836:string)
                              }
                            }
                            n397 = Concatenate Strings(w817, w814) -> (w815:string)
                            n398 = property class="Str"(reference=w825, error in=w808, "Text.Text"=w815) -> (error out=w810:errorcluster)  [unwired: 1 out]
                          }
                          frame "Units" {
                            n399 = disable-structure shown="Enabled" {
                              disable-tunnel: w845 -> [w858 _]
                              disable-tunnel: w844 -> [w855 _]
                              disable-tunnel: w843 -> [w853 _]
                              disable-tunnel: [w849 _] -> w842
                              disable-tunnel: w841 -> [w848 _]
                              disable-tunnel: w840 -> [w846 _]
                              frame Disabled {
                                w857 = refnum<vi> refnum  # String
                                n400 = Format Into String(DB_-_[Execute].[ActiveProcess]_Enum."[UnitOfTemperature]" ("[Execute].[ActiveProcess]\n2014-10-14 14:58")) -> (resulting string=w851:string)  [unwired: 3 in, 1 out]
                                n401 = Search 1D Array(1D array=w853, element=w851) -> (index of element=w850:i32)  [unwired: 1 in]
                                n402 = To More Specific Class(target class=w857, reference=w858, error in=w848) -> (specific class reference=w856:refnum<vi>, error out=w847:errorcluster)
                                n403 = Index Array(array=w855, index=w850) -> (element=w854:string)
                                n404 = property class="Str"(reference=w856, error in=w847, "Text.Text"=w854, "Text.BG Color"=w846) -> (error out=w849:errorcluster)  [unwired: 1 out]
                              }
                              frame Enabled {
                                # "Units now updated together with Temperature\nso the control item may not longer be needed"
                              }
                            }
                          }
                          frame "Alarm" {
                            w869 = refnum<vi> refnum  # String
                            n405 = Format Into String(DB_-_[Execute].[ActiveProcess]_Enum."[Message1]" ("[Execute].[ActiveProcess]\n2014-10-14 14:58")) -> (resulting string=w863:string)  [unwired: 3 in, 1 out]
                            n406 = Search 1D Array(1D array=w861, element=w863) -> (index of element=w862:i32)  [unwired: 1 in]
                            n407 = To More Specific Class(target class=w869, reference=w870, error in=w866) -> (specific class reference=w868:refnum<vi>, error out=w865:errorcluster)
                            n408 = Index Array(array=w860, index=w862) -> (element=w859:string)
                            n409 = property class="Str"(reference=w868, error in=w865, "Text.Text"=w859) -> (error out=w867:errorcluster)  [unwired: 1 out]
                          }
                          frame "% Hold Complete" {
                            w874 = refnum<vi> refnum  # NumericWithScale
                            n410 = Format Into String(DB_-_[Execute].[ActiveProcess]_Enum."[HoldTimePercentage]" ("[Execute].[ActiveProcess]\n2014-10-14 14:58")) -> (resulting string=w880:string)  [unwired: 3 in, 1 out]
                            n411 = Search 1D Array(1D array=w877, element=w880) -> (index of element=w879:i32)  [unwired: 1 in]
                            n412 = To More Specific Class(target class=w874, reference=w883, error in=w872) -> (specific class reference=w882:refnum<vi>, error out=w871:errorcluster)
                            n413 = Index Array(array=w878, index=w879) -> (element=w875:string)
                            n414 = Decimal String To Number(string=w875) -> (number=w876:i32)  [unwired: 2 in, 1 out]
                            n415 = property class="NumWthScl"(reference=w882, error in=w871, "Value"=w876) -> (error out=w873:errorcluster)  [unwired: 1 out]
                          }
                          frame "Temperature" {
                            w900 = "%_4f"  # 4 signficant Digits
                            w913 = refnum<vi> refnum  # String
                            n416 = Format Into String(DB_-_[Execute].[ActiveProcess]_Enum."[UnitOfTemperature]" ("[Execute].[ActiveProcess]\n2014-10-14 14:58")) -> (resulting string=w904:string)  [unwired: 3 in, 1 out]
                            n417 = Format Into String(DB_-_[Execute].[ActiveProcess]_Enum."[CurrentTemp]" ("[Execute].[ActiveProcess]\n2014-10-14 14:58")) -> (resulting string=w911:string)  [unwired: 3 in, 1 out]
                            n418 = Format Into String(DB_-_[Execute].[ActiveProcess]_Enum."[ControllerColor]" ("[Execute].[ActiveProcess]\n2014-10-14 14:58")) -> (resulting string=w890:string)  [unwired: 3 in, 1 out]
                            n419 = Search 1D Array(1D array=w892, element=w911) -> (index of element=w910:i32)  [unwired: 1 in]
                            n420 = Search 1D Array(1D array=w892, element=w904) -> (index of element=w903:i32)  [unwired: 1 in]
                            n421 = Search 1D Array(1D array=w892, element=w890) -> (index of element=w889:i32)  [unwired: 1 in]
                            n422 = To More Specific Class(target class=w913, reference=w915, error in=w907) -> (specific class reference=w914:refnum<vi>, error out=w906:errorcluster)
                            n423 = Index Array(array=w909, index #1=w910, index #2=w903, index #3=w889) -> (element #1=w899:string, element #2=w902:string, element #3=w888:string)
                            n424 = Fract/Exp String To Number(string=w899) -> (number=w898:dbl)  [unwired: 3 in, 1 out]
                            n425 = call <vilib>:"Space Constant.vi"() -> ("String"=w901:string)
                            n426 = Decimal String To Number(string=w888) -> (number=w885:i32)  [unwired: 2 in, 1 out]
                            n427 = Format Into String(format string=w900, w898) -> (resulting string=w897:string)  [unwired: 2 in, 1 out]
                            n428 = Concatenate Strings(w897, w901, w902) -> (w894:string)
                            n429 = Less Or Equal To 0?(x=w885) -> (x <= 0?=w887:bool)
                            n430 = Select(t="", s=w896, f=w894) -> (s? t:f=w893:string)
                            n431 = Select(t=u32 16777216, s=w887, f=w885) -> (s? t:f=w884:u32)
                            n432 = property class="Str"(reference=w914, error in=w906, "Value"=w893, "Text.BGColor"=w884) -> (error out=w908:errorcluster)  [unwired: 1 out]
                          }
                          frame "Graph" {
                            w934 = refnum<vi> refnum  # WaveformGraph
                            # "Row1, Column1"
                            n433 = call "DB - [CMS].[Execute].[ActiveProcess].vi"("Application"="CMS", "[PlantId],[SystemId]"=w920, "error in (no error)"=w930, "DB - CMS Execute ActiveProcess"=T24."SELECT FILESTREAM" ("DB - Execute ActiveProcess")) -> ("String ([RawDataFile] Filestream)"=w929:string, "SUMMARY"=w931:errorcluster)  [unwired: 12 in, 2 out]
                            n434 = local write "DB"(w931) -> ()
                            n435 = To More Specific Class(target class=w934, reference=w935, error in=w918) -> (specific class reference=w933:refnum<vi>, error out=w917:errorcluster)
                            n436 = Spreadsheet String To Array(delimiter (Tab)=",", format string="", spreadsheet string=w929, array type (2D Dbl)=dbl[][] []) -> (array=w925:dbl[][])
                            n437 = Array Subset(array=w925, index (row)=1 ("index"), index (col)=1 ("index")) -> (w922:dbl[][])  [unwired: 2 in]
                            n438 = Transpose 2D Array(2D array=w922) -> (transposed array=w921:dbl[][])
                            n439 = property class="WFGraph"(reference=w933, error in=w917, "Value"=w921) -> (error out=w919:errorcluster)  [unwired: 1 out]
                          }
                          frame "Last Updated On" {
                            w954 = refnum<vi> refnum  # String
                            n440 = To More Specific Class(target class=w954, reference=w953, error in=w945) -> (specific class reference=w955:refnum<vi>, error out=w944:errorcluster)
                            n441 = Format Into String(DB_-_[Execute].[ActiveProcess]_Enum."[LastUpdatedOn]" ("[Execute].[ActiveProcess]\n2014-10-14 14:58")) -> (resulting string=w950:string)  [unwired: 3 in, 1 out]
                            n442 = Search 1D Array(1D array=w949, element=w950) -> (index of element=w951:i32)  [unwired: 1 in]
                            n443 = Index Array(array=w948, index=w951) -> (element=w940:string)
                            n444 = Empty String/Path?(string/path=w940) -> (empty?=w939:bool)
                            n445 = call "String - Convert Str (YYYY-mm-dd HHcMMcSS) to TimeStamp.vi"("YYYY-mm-dd HH:MM:SS (String)"=w940) -> ("time stamp"=w941:timestamp)  [unwired: 9 in, 1 out]
                            n446 = Format Date/Time String(time format string (%c)=w947, seconds (now)=w941) -> (date/time string=w942:string)  [unwired: 1 in]
                            n447 = Concatenate Strings("last updated: " ("string"), w942) -> (w937:string)
                            n448 = Select(t="", s=w939, f=w937) -> (s? t:f=w936:string)
                            n449 = property class="Str"(reference=w955, error in=w944, "Value"=w936) -> (error out=w946:errorcluster)  [unwired: 1 out]
                          }
                          frame "Last Updated (Local)" {
                            w979 = refnum<vi> refnum  # String
                            n450 = Unbundle By Name(w969) -> ("PlantID"=w972:string, "SystemID"=w970:string)
                            n451 = Concatenate Strings(w972, "." ("string"), w970) -> (w962:string)
                            n452 = To More Specific Class(target class=w979, reference=w978, error in=w975) -> (specific class reference=w980:refnum<vi>, error out=w974:errorcluster)
                            n453 = Index Array(array="PlantId.SystemId - Last Updated (Local)", index (col)=0 ("disabled index (col)")) -> (element=w967:string[])  [unwired: 1 in]
                            n454 = Search 1D Array(1D array=w967, element=w962) -> (index of element=w966:i32)  [unwired: 1 in]
                            n455 = Format Date/Time String(time format string (%c)=w977, seconds (now)=w961) -> (date/time string=w964:string)  [unwired: 1 in]
                            n456 = case shown="-1" w966 {
                              selector: w966 -> [w984 _]
                              tunnel: "PlantId.SystemId - Last Updated (Local)" -> [w985 w990]
                              tunnel: w964 -> [w982 w988]
                              tunnel: [w981 w986] -> w963
                              tunnel: w962 -> [_ w989]
                              frame 0, Default {
                                # "Replace Last Updated (Local)"
                                n457 = Replace Array Subset(array=w985, new element=w982, index (row)=w984, index (col)=1 ("disabled index (col)")) -> (w981:string[][])
                              }
                              frame -1 {
                                # "Add Rrecord"
                                n458 = Build Array(w989, w988) -> (w987:string[])
                                n459 = Build Array (concatenate)(w990, w987) -> (w986:string[][])
                              }
                            }
                            n460 = local write "PlantId.SystemId - Last Updated (Local)"(w963) -> ()
                            n461 = Less?(x=w961, y=timestamp(3471350400 s since 1904-01-01)) -> (x < y?=w959:bool)
                            n462 = Concatenate Strings("last updated (local): " ("string"), w964) -> (w957:string)
                            n463 = Select(t="", s=w959, f=w957) -> (s? t:f=w956:string)
                            n464 = property class="Str"(reference=w980, error in=w974, "Value"=w956) -> (error out=w976:errorcluster)  [unwired: 1 out]
                          }
                          frame "Current Window" {
                            w1000 = refnum<vi> refnum  # Boolean
                            n465 = for {
                              tunnel: w997 -> [w1011] mode=indexing
                              tunnel: w996 -> [w1009]
                              tunnel: [w1004] -> w995
                              tunnel: w991 -> [w1001]
                              w1008 = refnum<vi> refnum  # Boolean
                              # "Set ALL WIN to FALSE"
                              n466 = property class="Clust (strict)"(reference=w1011, error in=w1001) -> (error out=w1003:errorcluster, "Controls[]"=w1010:refnum<vi>[])  [unwired: 1 out]
                              n467 = Index Array(array=w1010, index=w1009) -> (element=w1007:refnum<vi>)
                              n468 = To More Specific Class(target class=w1008, reference=w1007, error in=w1003) -> (specific class reference=w1006:refnum<vi>, error out=w1002:errorcluster)
                              n469 = property class="Bool"(reference=w1006, error in=w1002, "Value"=FALSE) -> (error out=w1004:errorcluster)  [unwired: 1 out]
                            }
                            n470 = To More Specific Class(target class=w1000, reference=w999, error in=w995) -> (specific class reference=w998:refnum<vi>, error out=w992:errorcluster)
                            n471 = property class="Bool"(reference=w998, error in=w992, "Value"=TRUE) -> (error out=w993:errorcluster)  [unwired: 1 out]
                          }
                        }
                        n472 = local write "Property Node"(w730) -> ()
                      }
                    }
                  }
                }
                frame False {
                  # "NotActive AND >60min"
                  n473 = property class="Clust (strict)"(reference=w1016) -> ("Controls[]"=w1018:refnum<vi>[])  [unwired: 1 in, 2 out]
                  n474 = case shown="\"WIN4\", \"WIN8\"" w1014 {
                    tunnel: w1018 -> [_ w1056]
                    tunnel: w1017 -> [_ w1055]
                    tunnel: w1015 -> [_ w1054]
                    frame "WIN1", Default {
                      w1021 = ""
                      w1034 = u32 10263708
                      n475 = local read "Skip WIN Timer"() -> (w1019:bool)
                      n476 = case shown="True" w1019 {
                        frame False {
                          # "Skip Timer"
                          n477 = local write "Skip Timer Count"(0 ("Skip Timer Count")) -> ()
                          n478 = local write "Skip WIN Timer"(TRUE ("Skip Timer")) -> ()
                        }
                        frame True {
                          # "Out of 24 Max"
                          # "Check if Skipped for 24 Times which implies no active Winxx"
                          n479 = local read "Skip Timer Count"() -> (w1039:i32)
                          n480 = for {
                            N: 24 -> [_]
                            tunnel: [w1046] -> w1042 mode=indexing if=w1044
                            i -> [w1048]
                            n481 = local read "Current WindowView"() -> (w1050:string[])
                            n482 = Add(x=DB_-_Config_WindowView_Enum."w.[Window01]", y=w1048) -> (x+y=w1047:i32)
                            n483 = Index Array(array=w1050, index=w1047) -> (element=w1046:string)
                            n484 = Empty String/Path?(string/path=w1046) -> (empty?=w1045:bool)
                            n485 = Not(x=w1045) -> (.not. x?=w1044:bool)
                          }
                          n486 = Increment(x=w1039) -> (x+1=w1038:i32)
                          n487 = local write "Skip Timer Count"(w1038) -> ()
                          n488 = Array Size(array=w1042) -> (size(s)=w1041:i32)
                          "# of requested Windowxx" <- w1041
                          n489 = Greater Or Equal?(x=w1038, y=w1041) -> (x >= y?=w1043:bool)
                          n490 = case shown="True" w1043 {
                            frame False {
                            }
                            frame True {
                              n491 = local write "Skip TAB Timer"(TRUE ("Skip TAB Timer")) -> ()
                            }
                          }
                        }
                      }
                      n492 = local write "Transaction No (Execute)"(w1021) -> ()
                      n493 = local write "WIN1 Bay"(w1021) -> ()
                      n494 = local write "TransactionRunNo (Execute)"(w1021) -> ()
                      n495 = local write "Key Values"(T4 {"Recording Duration"=0.0, "Remaining Hold Time"=0.0, "Current Temp"=0.0, "Key Values Temperature Units"=""} ("Key Values")) -> ()
                      n496 = local write "% Hold. Time Completed"(0.0 ("% Hold. Time Completed")) -> ()
                      n497 = local write "Sequence Status"("") -> ()
                      n498 = property on="cRIO Status" class="Str"("Text.BG Color"=u32 16777216, "Text.Text"="") -> ()  [unwired: 2 in, 2 out]
                      n499 = property on="ET3504 Status" class="Str"("Text.BG Color"=u32 16777216, "Text.Text"="") -> ()  [unwired: 2 in, 2 out]
                      n500 = Bundle(w1034, w1034) -> (w1035:cluster{u32, u32})  [unwired: 1 in]
                      n501 = Build Array(w1035, w1035) -> (w1033:cluster{u32, u32}[])
                      n502 = property on="Process Completed" class="Bool (strict)"("Colors [4]"=w1033) -> (error out=w1031:errorcluster)  [unwired: 2 in, 1 out]
                      n503 = property on="Overall Status" class="Bool (strict)"("Colors [4]"=w1033) -> (error out=w1030:errorcluster)  [unwired: 2 in, 1 out]
                      n504 = property on="Hold Time Completed" class="Bool (strict)"("Colors [4]"=w1033) -> (error out=w1032:errorcluster)  [unwired: 2 in, 1 out]
                      n505 = property on="% Hold. Time Completed" class="Slide (strict)"("Fill Color"=u32 16777216) -> ()  [unwired: 2 in, 2 out]
                      n506 = Merge Errors(w1032, w1031, w1030) -> (w1029:errorcluster)
                      n507 = local write "Property Node"(w1029) -> ()
                    }
                    frame "WIN4", "WIN8" {
                      # "Reset Skip Timer"
                      n508 = for {
                        tunnel: w1056 -> [w1064] mode=indexing
                        tunnel: w1055 -> [w1061]
                        tunnel: w1054 -> [w1060]
                        i -> [w1059]
                        n509 = property class="Ctl"(reference=w1064) -> (reference out=w1063:refnum<vi>, error out=w1057:errorcluster, "Label.Text"=w1062:string)  [unwired: 1 in]
                        n510 = case shown="\"Last Updated (Local)\"" w1062 {
                          tunnel: w1063 -> [w1070 w1088 w1102 w1109 w1116 w1123 w1130 w1137 w1144 w1151 w1155 w1166]
                          tunnel: w1061 -> [w1066 w1079 _ _ _ _ _ _ _ _ _ _]
                          tunnel: w1060 -> [_ _ _ _ _ _ _ _ _ _ _ w1164]
                          tunnel: w1059 -> [_ _ _ _ _ _ _ _ _ _ _ w1163]
                          tunnel: [w1069 w1087 w1096 w1103 w1110 w1117 w1124 w1131 w1138 w1145 w1152 w1159] -> w1058
                          tunnel: w1057 -> [w1068 w1086 w1098 w1105 w1112 w1119 w1126 w1133 w1140 w1147 w1154 w1162]
                          frame "Bay", Default {
                            w1072 = refnum<vi> refnum  # String
                            n511 = Unbundle By Name(w1066) -> ("SystemID"=w1065:string)
                            n512 = To More Specific Class(target class=w1072, reference=w1070, error in=w1068) -> (specific class reference=w1071:refnum<vi>, error out=w1067:errorcluster)
                            n513 = property class="Str"(reference=w1071, error in=w1067, "Value"=w1065) -> (error out=w1069:errorcluster)  [unwired: 1 out]
                          }
                          frame "Last Updated (Local)" {
                            w1077 = 0  # PlantId.SystemId
                            w1085 = refnum<vi> refnum  # String
                            n514 = local read "PlantId.SystemId - Last Updated (Local)"() -> (w1074:string[][])
                            n515 = Unbundle By Name(w1079) -> ("PlantID"=w1082:string, "SystemID"=w1080:string)
                            n516 = Concatenate Strings(w1082, "." ("string"), w1080) -> (w1078:string)
                            n517 = Index Array(array=w1074, index (col)=w1077) -> (element=w1076:string[])  [unwired: 1 in]
                            n518 = To More Specific Class(target class=w1085, reference=w1088, error in=w1086) -> (specific class reference=w1084:refnum<vi>, error out=w1083:errorcluster)
                            n519 = Search 1D Array(1D array=w1076, element=w1078) -> (index of element=w1075:i32)  [unwired: 1 in]
                            n520 = case shown="0, Default" w1075 {
                              selector: w1075 -> [w1093 _]
                              tunnel: w1074 -> [w1094 _]
                              tunnel: [w1089 "" ("String")] -> w1073
                              frame 0, Default {
                                w1092 = 1  # Last Updated (Local)
                                # "Found"
                                n521 = Index Array(array=w1094, index (row)=w1093, index (col)=w1092) -> (element=w1090:string)
                                n522 = Concatenate Strings("last updated (local): " ("string"), w1090) -> (w1089:string)
                              }
                              frame -1 {
                                # "Not Found"
                              }
                            }
                            n523 = property class="Str"(reference=w1084, error in=w1083, "Value"=w1073) -> (error out=w1087:errorcluster)  [unwired: 1 out]
                          }
                          frame "Seq Status" {
                            w1101 = refnum<vi> refnum  # String
                            n524 = To More Specific Class(target class=w1101, reference=w1102, error in=w1098) -> (specific class reference=w1100:refnum<vi>, error out=w1097:errorcluster)
                            n525 = property class="Str"(reference=w1100, error in=w1097, "Text.Text"="Waiting to Start") -> (error out=w1096:errorcluster)  [unwired: 1 out]
                          }
                          frame "Record" {
                            w1108 = refnum<vi> refnum  # String
                            n526 = To More Specific Class(target class=w1108, reference=w1109, error in=w1105) -> (specific class reference=w1107:refnum<vi>, error out=w1104:errorcluster)
                            n527 = property class="Str"(reference=w1107, error in=w1104, "Text.Text"="") -> (error out=w1103:errorcluster)  [unwired: 1 out]
                          }
                          frame "Hold" {
                            w1115 = refnum<vi> refnum  # String
                            n528 = To More Specific Class(target class=w1115, reference=w1116, error in=w1112) -> (specific class reference=w1114:refnum<vi>, error out=w1111:errorcluster)
                            n529 = property class="Str"(reference=w1114, error in=w1111, "Text.Text"="") -> (error out=w1110:errorcluster)  [unwired: 1 out]
                          }
                          frame "Units" {
                            w1122 = refnum<vi> refnum  # String
                            n530 = To More Specific Class(target class=w1122, reference=w1123, error in=w1119) -> (specific class reference=w1121:refnum<vi>, error out=w1118:errorcluster)
                            n531 = property class="Str"(reference=w1121, error in=w1118, "Text.Text"="") -> (error out=w1117:errorcluster)  [unwired: 1 out]
                          }
                          frame "Alarm" {
                            w1129 = refnum<vi> refnum  # String
                            n532 = To More Specific Class(target class=w1129, reference=w1130, error in=w1126) -> (specific class reference=w1128:refnum<vi>, error out=w1125:errorcluster)
                            n533 = property class="Str"(reference=w1128, error in=w1125, "Text.Text"="") -> (error out=w1124:errorcluster)  [unwired: 1 out]
                          }
                          frame "% Hold Complete" {
                            w1136 = refnum<vi> refnum  # NumericWithScale
                            n534 = To More Specific Class(target class=w1136, reference=w1137, error in=w1133) -> (specific class reference=w1135:refnum<vi>, error out=w1132:errorcluster)
                            n535 = property class="NumWthScl"(reference=w1135, error in=w1132, "Value"=0) -> (error out=w1131:errorcluster)  [unwired: 1 out]
                          }
                          frame "Temperature" {
                            w1143 = refnum<vi> refnum  # String
                            n536 = To More Specific Class(target class=w1143, reference=w1144, error in=w1140) -> (specific class reference=w1142:refnum<vi>, error out=w1139:errorcluster)
                            n537 = property class="Str"(reference=w1142, error in=w1139, "Value"="") -> (error out=w1138:errorcluster)  [unwired: 1 out]
                          }
                          frame "Graph" {
                            w1150 = refnum<vi> refnum  # WaveformGraph
                            n538 = To More Specific Class(target class=w1150, reference=w1151, error in=w1147) -> (specific class reference=w1149:refnum<vi>, error out=w1146:errorcluster)
                            n539 = property class="WFGraph"(reference=w1149, error in=w1146, "Value"=dbl[][] []) -> (error out=w1145:errorcluster)  [unwired: 1 out]
                          }
                          frame "Last Updated On" {
                            w1158 = refnum<vi> refnum  # String
                            n540 = To More Specific Class(target class=w1158, reference=w1155, error in=w1154) -> (specific class reference=w1157:refnum<vi>, error out=w1153:errorcluster)
                            n541 = property class="Str"(reference=w1157, error in=w1153, "Value"="") -> (error out=w1152:errorcluster)  [unwired: 1 out]
                          }
                          frame "Current Window" {
                            w1168 = refnum<vi> refnum  # Boolean
                            n542 = for {
                              tunnel: w1164 -> [w1177] mode=indexing
                              tunnel: w1163 -> [w1175]
                              tunnel: [w1170] -> w1161
                              tunnel: w1162 -> [w1169]
                              w1174 = refnum<vi> refnum  # Boolean
                              n543 = property class="Clust (strict)"(reference=w1177, error in=w1169) -> ("Controls[]"=w1176:refnum<vi>[])  [unwired: 2 out]
                              n544 = Index Array(array=w1176, index=w1175) -> (element=w1173:refnum<vi>)
                              n545 = To More Specific Class(target class=w1174, reference=w1173) -> (specific class reference=w1172:refnum<vi>)  [unwired: 1 in, 1 out]
                              n546 = property class="Bool"(reference=w1172, "Value"=FALSE) -> (error out=w1170:errorcluster)  [unwired: 1 in, 1 out]
                            }
                            n547 = To More Specific Class(target class=w1168, reference=w1166, error in=w1161) -> (specific class reference=w1167:refnum<vi>, error out=w1160:errorcluster)
                            n548 = property class="Bool"(reference=w1167, error in=w1160, "Value"=TRUE) -> (error out=w1159:errorcluster)  [unwired: 1 out]
                          }
                        }
                        n549 = local write "Property Node"(w1058) -> ()
                      }
                      n550 = local write "Skip WIN Timer"(FALSE ("Skip Timer")) -> ()
                      n551 = local write "Skip Timer Count"(0 ("Skip Timer Count")) -> ()
                    }
                  }
                }
              }
            }
          }
          n552 = local read "Logon OK"() -> (w312:bool)
          n553 = local read "Close Flag"() -> (w315:bool)
          n554 = Not(x=w312) -> (.not. x?=w314:bool)
          n555 = Or(x=w314, y=w315) -> (x .or. y?=w313:bool)
          n556 = Select "Check if User Log off"(t=w311, s=w312, f=w309) -> (s? t:f=w310:T10)
        }
      }
      frame "QUIT" {
      }
    }
    n557 = Wait Until Next ms Multiple(millisecond multiple=u32 100) -> ()  [unwired: 1 out]
    n558 = Format Date/Time String(time format string (%c)="%b %d, %Y  %H:%M:%S") -> (date/time string=→"Date Time":string)  [unwired: 2 in]
    n559 = local read "Quit Flag"() -> (w117:bool)
    n560 = Select(t=w116, s=w117, f=w114) -> (s? t:f=w115:T10)
  }
  n561 = while {
    tunnel: w4 -> [_]
    tunnel: [w1180] -> w1
    stop <- w1180 stop-if-true
    # "Event Structure For UIEvents"
    n562 = event shown="[2] \"Cluster0 WIN8\", \"Cluster1 WIN8\", \"Cluster2 WIN8\", \"Cluster3 WIN8\", \"Cluster4 WIN8\", \"Cluster6 WIN8\", \"Cluster7 WIN8\", \"Cluster0 WIN4\", \"Cluster1 WIN4\", \"Cluster2 WIN4\", \"Cluster3 WIN4\", \"Cluster5 WIN8\": Mouse Down" {
      selector: _ -> [_ _ _ _ _ _]
      dyn-events: _ -> [_ _ _ _ _ _]
      timeout: _ -> [_ _ _ _ _ _]
      tunnel: [_ _ _ w1270 _ _] -> _
      tunnel: [_ _ _ w1269 _ _] -> w1180
      event Timeout {
        n563 = event-data() -> ()  [unwired: 1 in, 3 out]
      }
      event "Tab Body": Value Change {
        n564 = event-data() -> ("NewVal"=w1181:T1)  [unwired: 1 in, 5 out]
        n565 = case shown="\"Admin\"..\"Logon\"" w1181 {
          selector: w1181 -> [w1186 _]
          frame "Admin".."Logon" {
            # "Enable ToggleTab Override"
            # "SubPanel VI's Path\n..\\SRTRS\\VIs\\SubPanels\\DB UI - Logon.vi\nOR \n..\\SRTRS\\MyEXE.exe\\SubPanels\\DB UI - Logon.vi"
            # "Current VI's Path\n..\\SRTRS\\VIs\\Main.vi\nOR \n..\\SRTRS\\MyEXE.exe\\Main.vi"
            n566 = case shown="\"Logon\"" w1186 {
              tunnel: [w1231 w1233 w1237] -> w1187
              tunnel: ["DB UI - Config.vi" ("name or relative path") "DB UI - Logon.vi" ("name or relative path") "DB UI - Admin User.vi" ("name or relative path")] -> w1185
              frame "Config", Default {
                # "Config"
                n567 = control-ref of="Config UI"() -> (w1231:refnum<vi>)
              }
              frame "Logon" {
                n568 = control-ref of="Logon UI"() -> (w1233:refnum<vi>)
                n569 = property on="Close" class="Bool (strict)"("BoolText.Text"="Close") -> ()  [unwired: 2 in, 2 out]
              }
              frame "Admin" {
                # "User or Equipment CHILD TAB"
                n570 = control-ref of="Admin User UI"() -> (w1237:refnum<vi>)
              }
            }
            n571 = local read "Current VI's path"() -> (w1194:path)
            n572 = Strip Path(path=w1194) -> (stripped path=w1197:path)  [unwired: 1 out]
            n573 = Build Path(base path=w1197, name or relative path="SubPanels") -> (appended path=w1195:path)
            n574 = Build Path(base path=w1195, name or relative path=w1185) -> (appended path=w1191:path)
            n575 = Open VI Reference(vi path=w1191, error in (no error)=errorcluster {"status"=FALSE, "code"=0, "source"=""}) -> (vi reference=w1193:refnum<vi>, error out=w1188:errorcluster)  [unwired: 4 in]
            n576 = case shown="\"Logon\"" w1186 {
              tunnel: w1193 -> [w1228 w1229 w1230]
              frame "Config", Default {
                # "Config"
                "Config UI" <- w1228
              }
              frame "Logon" {
                "Logon UI" <- w1229
              }
              frame "Admin" {
                # "User or Equipment CHILD TAB"
                "Admin User UI" <- w1230
              }
            }
            n577 = property class="VI"(reference=w1193) -> (reference out=w1189:refnum<vi>, "Exec.State"=w1190:T9, "FP.State"=→"Front Panel Window:State":T8)  [unwired: 1 in, 1 out]
            "Execution:State" <- w1190
            n578 = local write "[ToggleTab] Override"(TRUE ("[ToggleTab] Override")) -> ()
            n579 = case shown="\"Idle\"" w1190 {
              tunnel: w1188 -> [w1199 w1221]
              tunnel: [w1198 w1219] -> w1182
              tunnel: w1189 -> [w1200 w1214]
              tunnel: ["UI Already Loaded" ("string") " UI Load OK." ("string")] -> _
              tunnel: w1187 -> [_ w1212]
              tunnel: w1186 -> [_ w1206]
              frame "Running", Default {
                # "Close Each time to release the Ref.\nA new Ref will be created each time use Changes\nTab. No problem here because VI still Running."
                # "Already Running"
                n580 = Close Reference(reference=w1200, error in (no error)=w1199) -> (error out=w1198:errorcluster)
              }
              frame "Idle" {
                w1217 = T11."Off While Running" ("Horizontal Scrollbar Visibility")
                # "Panel Size not Writable only Readable"
                # "Not Running YET"
                n581 = property class="VI"(reference=w1214, error in=w1221) -> (error out=w1220:errorcluster, "Panel"=w1222:refnum<vi>)  [unwired: 1 out]
                n582 = property class="Pnl"(reference=w1222, error in=w1220) -> (error out=w1205:errorcluster, "Panes[]"=w1207:refnum<vi>[], "Controls[]"=w1204:refnum<vi>[])  [unwired: 1 out]
                n583 = case shown="\"Admin\"..\"Logon\"" w1206 {
                  tunnel: w1204 -> [_ w1224]
                  tunnel: [w1223 w1226] -> w1203
                  tunnel: w1205 -> [w1223 w1225]
                  frame "WIN8", Default {
                  }
                  frame "Admin".."Logon" {
                    n584 = control-ref of="Application"() -> (w1227:refnum<vi>)
                    n585 = call "subPanel - Write Value.vi"("Error In"=w1225, "CtlRef Controls[]"=w1224, "Pnl Control"=w1227) -> ("Error Out"=w1226:errorcluster)  [unwired: 6 in, 2 out]
                  }
                }
                n586 = Index Array(array=w1207, index=0) -> (element=w1215:refnum<vi>)
                n587 = property class="Pane"(reference=w1215, error in=w1203, "HorizScrollbarVisibility"=w1217, "VertScrollbarVisibility"=w1217, "Origin"=T13 {"Horizontal"=0, "Vertical"=0}) -> (error out=w1202:errorcluster)  [unwired: 1 out]
                n588 = invoke class="VI" method="Run VI"(reference=w1214, error in=w1202, "Wait until done"=FALSE ("Wait Until Done"), "Auto Dispose Ref"=FALSE ("Auto Dispose Reference")) -> (reference out=w1208:refnum<vi>, error out=w1209:errorcluster)  [unwired: 1 in, 3 out]
                n589 = invoke on="Invoke Node" class="SubPnl" method="Insert VI"(reference=w1212, error in=w1209, "VI Ref"=w1208) -> (error out=w1219:errorcluster)  [unwired: 1 in, 3 out]
              }
            }
            "SubPanel Error" <- w1182
          }
          frame Default {
            # "Toggle Overide once user clicks on any TAB\n[Set [ToggleTab] Override = True\nSET Stay in [WINDOWxx] = False \n Continue to Toggle between WINDOWs starting from this Tab"
            n590 = local read "WindowView (ORDERed by DB)"() -> (w1246:string[][])
            n591 = local read "Tab Body"() -> (w1242:T1)
            n592 = property on="Tab Body" class="TabCtl (strict)"() -> ("Pages"=w1243:refnum<vi>[])  [unwired: 2 in, 2 out]
            n593 = Index Array(array=w1243, index=w1242) -> (element=w1241:refnum<vi>)
            n594 = property class="Page"(reference=w1241) -> ("PageLabel"=w1240:string)  [unwired: 1 in, 2 out]
            "Page Label when Menu is Clicked" <- w1240
            n595 = Index Array(array=w1246, index (col)=0 ("disabled index (col)")) -> (element=w1244:string[])  [unwired: 1 in]
            n596 = local write "Stay in [WINDOWxx]"(FALSE ("Stay in [WINDOWxx]")) -> ()
            n597 = local write "[ToggleTab] Override"(TRUE ("[ToggleTab] Override")) -> ()
            n598 = Search 1D Array(1D array=w1244, element=w1240) -> (index of element=w1239:i32)  [unwired: 1 in]
            n599 = flat-sequence {
              tunnel: w1239 -> [w1248]
              frame #0 {
                "New [TabId] Index" <- w1248
              }
              frame #1 {
                n600 = local write "Reset [TabId] Index"(TRUE ("Reset [TabId] Index")) -> ()
              }
            }
          }
        }
      }
      event Mouse Down {
        # "USER Clicks on any of the WIN8 or WIN4 Windows\nSet to WIN1 and \nSET Stay in [WINDOWxx]  in current [WINDOWxx]\n SET [ToggleTabInterval] Override = True"
        n601 = event-data() -> ("Time"=→"Time (WIN8 Click)":u32, "CtlRef"=w1251:refnum<vi>, "Mods.Double Click"=w1250:bool)  [unwired: 1 in, 5 out]
        n602 = case shown="True" w1250 {
          tunnel: w1251 -> [_ w1255]
          frame False {
          }
          frame True {
            w1256 = "WIN1" ("Page Label when Menu is Clicked")
            n603 = property class="Clust (strict)"(reference=w1255) -> ("Value"=w1253:T3)  [unwired: 1 in, 2 out]
            n604 = Unbundle By Name(w1253) -> ("[PlantId.SystemId]"=→"[WINDOWxx] Stay":string)
            n605 = local read "WindowView (ORDERed by DB)"() -> (w1261:string[][])
            n606 = local write "Page Label when Menu is Clicked"(w1256) -> ()
            n607 = local write "[ToggleTab] Override"(TRUE ("[ToggleTab] Override")) -> ()
            n608 = local write "Stay in [WINDOWxx]"(TRUE ("Stay in [WINDOWxx]")) -> ()
            n609 = Index Array(array=w1261, index (col)=0 ("disabled index (col)")) -> (element=w1259:string[])  [unwired: 1 in]
            n610 = local write "Tab Body"(CMS_Windows_Tab."WIN1" ("Tab Body")) -> ()
            n611 = Search 1D Array(1D array=w1259, element=w1256) -> (index of element=w1258:i32)  [unwired: 1 in]
            n612 = flat-sequence {
              tunnel: w1258 -> [w1264]
              frame #0 {
                n613 = local write "New [TabId] Index"(w1264) -> ()
              }
              frame #1 {
                n614 = local write "Reset [TabId] Index"(TRUE ("Reset [TabId] Index")) -> ()
              }
            }
          }
        }
      }
      event "Close", "Debug Close": Value Change {
        n615 = event-data() -> ("NewVal"=w1270:bool)  [unwired: 1 in, 5 out]
        n616 = local read "Show Debug TAB"() -> (w1268:bool)
        n617 = And(x=w1268, y="Debug Close") -> (x .and. y?=w1266:bool)
        n618 = case shown="False" w1266 {
          tunnel: [w1272 w1344] -> w1269
          frame False {
            # "Close OR Log off"
            n619 = property on="Close" class="Bool (strict)"() -> ("BoolText.Text"=w1271:string)  [unwired: 2 in, 2 out]
            n620 = case shown="\"Log off\", Default" w1271 {
              tunnel: [FALSE ("T button?") w1335] -> w1272
              frame "Log off", Default {
                n621 = First Call?() -> (First Call?: T/F=w1274:bool)
                n622 = case shown="False" w1274 {
                  tunnel: [w1279 TRUE ("T button?")] -> w1275
                  frame False {
                    # "Prompt on subsequent Log off"
                    n623 = call "Msgbox - Message Handler.vi"("Application (Default SRTRS)"="CMS", "Short Description (When DB Not Available)"="Log off Application.", "Description (When DB Not Available)"="All unsaved data will be lost. Do you want to proceed Logoff?", "<.?....> Message Code"="<W 001>") -> ("MHandler Error"=→"MHandler":errorcluster, "OK Out"=w1279:bool)  [unwired: 5 in, 1 out]
                  }
                  frame True {
                    (unwired) "1st Startup." ("string")
                    # "1st Startup, no prompt"
                  }
                }
                n624 = local write "Close"(FALSE ("Quit")) -> ()
                n625 = case shown="True" w1275 {
                  frame False {
                  }
                  frame True {
                    # "Need to Stop\nthe {Running Process}\nLoop"
                    # "Log off CONFIRMED"
                    n626 = flat-sequence {
                      tunnel: [errorcluster {"status"=FALSE, "code"=0, "source"=""} ("error constant")] -> w1290
                      frame #0 {
                        w1331 = ""
                        n627 = local read "Plant and Furnace Name (B4 Logon)"() -> (w1325:string)
                        n628 = global read "Global CMS.vi" "Logon Extra"() -> (w1328:T6)
                        n629 = Bundle By Name(cluster=w1328, "UserName"=w1331) -> (w1327:T6)
                        n630 = global read "Global CMS.vi" "Logon"() -> (w1332:T7)
                        n631 = Bundle By Name(cluster=w1332, "UserID"=w1331) -> (w1329:T7)
                        n632 = local write "Plant and Furnace Name"(w1325) -> ()
                        n633 = local write "Logon OK"(FALSE ("Logon OK")) -> ()
                        n634 = global write "Global CMS.vi" "Logon Extra"(w1327) -> ()
                        n635 = global write "Global CMS.vi" "Logon"(w1329) -> ()
                      }
                    }
                    n636 = local read "Show Debug TAB"() -> (w1289:bool)
                    n637 = local read "Lite Version"() -> (w1288:bool)
                    n638 = local read "DB - Logon"() -> (w1287:bool)
                    n639 = property on="Tab Body" class="TabCtl (strict)"() -> ("Pages"=w1291:refnum<vi>[])  [unwired: 2 in, 2 out]
                    n640 = case shown="False" w1287 {
                      tunnel: w1289 -> [w1296 w1313]
                      tunnel: w1288 -> [w1295 _]
                      tunnel: w1291 -> [w1294 w1312]
                      tunnel: w1290 -> [w1293 w1310]
                      tunnel: [w1292 w1311] -> w1285
                      frame False {
                        # "No DB"
                        n641 = for {
                          tunnel: w1294 -> [w1305] mode=indexing
                          tunnel: w1296 -> [w1304]
                          tunnel: w1295 -> [w1301]
                          tunnel: w1293 -> [w1299]
                          tunnel: [w1298] -> w1292
                          (unwired) "Debug" ("y")
                          n642 = property class="Page"(reference=w1305, error in=w1299) -> (reference out=w1300:refnum<vi>, error out=w1297:errorcluster, "PageLabel"=w1303:string)
                          n643 = case shown="\"\"" w1303 {
                            tunnel: w1304 -> [_ w1308 _]
                            tunnel: [w1306 w1308 TRUE] -> w1302
                            tunnel: w1301 -> [w1307 _ _]
                            frame "" {
                              # "If Lite Version\nthese TAB will be hidden"
                              n644 = Not(x=w1307) -> (.not. x?=w1306:bool)
                            }
                            frame "Debug" {
                              # "Debug dependent of \n\"Show Debug Tab ONLY\""
                            }
                            frame Default {
                              # "These Tabs ALWAYS shown"
                            }
                          }
                          n645 = property class="Page"(reference=w1300, error in=w1297, "PageVis"=w1302) -> (error out=w1298:errorcluster)  [unwired: 1 out]
                        }
                      }
                      frame True {
                        # "Use DB to Logon"
                        n646 = for {
                          tunnel: w1312 -> [w1321] mode=indexing
                          tunnel: w1313 -> [w1320]
                          tunnel: [w1316] -> w1311
                          tunnel: w1310 -> [w1314]
                          (unwired) "Debug" ("y")
                          n647 = property class="Page"(reference=w1321, error in=w1314) -> (reference out=w1317:refnum<vi>, error out=w1315:errorcluster, "PageLabel"=w1319:string)
                          n648 = case shown="Default" w1319 {
                            tunnel: w1320 -> [_ w1323 _]
                            tunnel: [FALSE ("Show Debug Tab") w1323 TRUE] -> w1318
                            frame Default {
                              # "All\nthese TAB will be hidden"
                            }
                            frame "Debug" {
                              # "Show Debug?"
                            }
                            frame "Logon" {
                              # "These Tabs ALWAYS shown"
                            }
                          }
                          n649 = property class="Page"(reference=w1317, error in=w1315, "PageVis"=w1318) -> (error out=w1316:errorcluster)  [unwired: 1 out]
                        }
                      }
                    }
                    n650 = property on="Tab Body" class="TabCtl (strict)"(error in=w1285, "Val(Sgnl)"=CMS_Windows_Tab."Logon" ("Tab Body")) -> (error out=→"Error Out":errorcluster)  [unwired: 1 in, 1 out]
                  }
                }
              }
              frame "Close" {
                n651 = call "Msgbox - Message Handler.vi"("Application (Default SRTRS)"="CMS", "Short Description (When DB Not Available)"="Close Application", "Description (When DB Not Available)"="Confirm close Application?", "<.?....> Message Code"="<W 104>") -> ("MHandler Error"=w1334:errorcluster, "OK Out"=w1335:bool)  [unwired: 5 in, 1 out]
                n652 = local write "Quit Flag"(w1335) -> ()
                n653 = local write "MHandler"(w1334) -> ()
                n654 = flat-sequence {
                  tunnel: [w1341] -> w1340
                  tunnel: "Close" -> [w1341]
                  tunnel: w1340 -> [_]
                  frame #0 {
                    n655 = Wait (ms)(milliseconds to wait=u32 100) -> ()  [unwired: 1 out]
                  }
                  frame #1 {
                    n656 = local write "Close"(FALSE ("Quit")) -> ()
                  }
                }
              }
            }
          }
          frame True {
            # "Debug Close"
            n657 = flat-sequence {
              tunnel: [w1345] -> w1344
              frame #0 {
                w1345 = TRUE ("T button?")
                n658 = local write "Quit Flag"(w1345) -> ()
              }
              frame #1 {
                n659 = Wait Until Next ms Multiple(millisecond multiple=u32 200) -> ()  [unwired: 1 out]
              }
              frame #2 {
                n660 = disable-structure shown="Disabled" {
                  frame Disabled {
                    n661 = call "Msgbox - Format Message.vi"("Message"="{Debug CLOSE}" ("string"), "Message Code\n2014-10-01"=Message_Code_-_Enum."<APP><W 113>" ("Message Code\n2014-10-01")) -> ("Message"=w1347:string)  [unwired: 8 in, 1 out]
                    n662 = call "Queue - EnQueue to MessageQ.vi"("Message"=w1347) -> ()  [unwired: 10 in, 1 out]
                  }
                  frame Enabled {
                  }
                }
              }
            }
          }
        }
      }
      event "Tab Body": Shortcut Menu Selection (User) {
        n663 = event-data() -> ("ItemTag"=w1350:string)  [unwired: 1 in, 7 out]
        n664 = case shown="\"Toggle Between Tabs\"" w1350 {
          frame "False", Default {
          }
          frame "Toggle Between Tabs" {
            # "Enable/Disable [ToggleTab] Override"
            n665 = local read "[ToggleTab]"() -> (w1351:bool)
            n666 = case shown="True" w1351 {
              frame False {
              }
              frame True {
                # "Only allowed if [ToggleTab] is TRUE"
                n667 = local read "[ToggleTab] Override"() -> (w1354:bool)
                n668 = local write "Stay in [WINDOWxx]"(FALSE ("Stay in [WINDOWxx]")) -> ()
                n669 = Not(x=w1354) -> (.not. x?=w1352:bool)
                n670 = local write "[ToggleTab] Override"(w1352) -> ()
                n671 = disable-structure shown="Disabled" {
                  disable-tunnel: w1352 -> [w1362 _]
                  frame Disabled {
                    n672 = Select(t="Disabled.", s=w1362, f="Enabled.") -> (s? t:f=w1359:string)
                    n673 = Concatenate Strings("<I0000> Toggling Between Tabs is " ("Message IN"), w1359) -> (w1356:string)
                    n674 = call "tool_Unicode_Convert ASCII to Unicode (Scalar).vi"("ASCII"=w1356) -> ("Unicode"=w1355:string)  [unwired: 4 in]
                    n675 = call "Msgbox UI.vi"("<xxxxxx> + Pre+Description+Post (Unicode)"=w1355, "[MessageType]"="i") -> ()  [unwired: 7 in, 3 out]
                  }
                  frame Enabled {
                  }
                }
              }
            }
          }
        }
      }
      event "Tab Body": Shortcut Menu Activation? {
        w1368 = "Toggle Between Tabs" ("item tag")
        # "Allow user to Re-Enable [ToggleTab] \nif it was already disabled"
        n676 = event-data() -> ("MenuRef"=w1367:refnum<k9>)  [unwired: 1 in, 6 out]
        n677 = local read "[ToggleTab] Override"() -> (w1366:bool)
        n678 = local read "[ToggleTab]"() -> (w1363:bool)
        n679 = Not(x=w1366) -> (.not. x?=w1365:bool)
        n680 = And(x=w1365, y=w1363) -> (x .and. y?=w1364:bool)
        n681 = Set Menu Item Info(6:w1364, 7:w1368, 9:w1363, 10:w1368, 11:w1367) -> ()  [unwired: 2 in, 2 out]
        n682 = event-data() -> ()  [unwired: 2 in, 1 out]
      }
    }
    "Close Flag" <- w1180
  }
  n683 = flat-sequence {
    tunnel: w2 -> [_]
    tunnel: w1 -> [_]
    frame #0 {
      n684 = local read "Application:Name"() -> (w1374:string)
      n685 = To Upper Case(1:w1374) -> (0:w1373:string)
      n686 = To Upper Case(1:"LabVIEW.exe" ("regular expression")) -> (0:w1371:string)
      n687 = Match Pattern(string=w1373, regular expression=w1371) -> (offset past match=w1370:i32)  [unwired: 1 in, 3 out]
      n688 = Greater Or Equal To 0?(x=w1370) -> (x >= 0?=w1369:bool)
      n689 = case shown="True" w1369 {
        frame False {
          # "Executable"
          n690 = control-ref of="This VI"() -> (w1375:refnum<vi>)
          n691 = invoke class="VI" method="FP.Close"(reference=w1375) -> ()  [unwired: 2 in, 3 out]
        }
        frame True {
          # "Show Debug TAB"
          # "LabVIEW Development"
          n692 = property on="Tab Body" class="TabCtl (strict)"() -> ("Pages"=w1376:refnum<vi>[])  [unwired: 2 in, 2 out]
          n693 = for {
            tunnel: w1376 -> [w1381] mode=indexing
            n694 = property class="Page"(reference=w1381) -> (reference out=w1377:refnum<vi>, "PageLabel"=w1380:string)  [unwired: 1 in, 1 out]
            n695 = Equal?(x=w1380, y="Debug") -> (x = y?=w1378:bool)
            n696 = case shown="True" w1378 {
              tunnel: w1377 -> [_ w1383]
              frame False {
              }
              frame True {
                n697 = property class="Page"(reference=w1383, "PageVis"=TRUE) -> ()  [unwired: 1 in, 2 out]
              }
            }
          }
        }
      }
    }
  }
